vi "总磷总氮通讯.vi"() -> ()   [LabVIEW 2016, in "斯坦道总氮.lvlib"]
uses:
  <vilib>/Plasmionique/MB Master/MB_Master_Serial/MB_Master_Serial.lvclass
  C:/Program Files (x86)/National Instruments/LabVIEW 2016/vi.lib/Plasmionique/MB Master/MB_Master/MB_Master.lvclass
  <vilib>/Plasmionique/MB Master/MB_Master_TCP/MB_Master_TCP.lvclass
  <vilib>/Utility/config.llb/Write Key (Boolean).vi
  <vilib>/Utility/config.llb/Write Key (String).vi
  <vilib>/Plasmionique/MB Master/MB_Master/MB_Master.lvclass
  <vilib>/Utility/config.llb/NI_LVConfig.lvlib
  <vilib>/Plasmionique/MB Master/MB Master.lvlib
  <vilib>/ptbypt/NI_PtbyPt.lvlib
panel:
  out "启用":bool=TRUE
  out "氨氮状态告警区":u16[](array[numeric])
  out "氨氮测量数据区":u16[](array[numeric])
  out "COD测量数据区":u16[](array[numeric])
  out "COD状态告警区":u16[](array[numeric])
  out "总氮测量数据区":u16[](array[numeric])
  out "总氮状态告警区":u16[](array[numeric])
  out "总磷状态告警区":u16[](array[numeric])
  out "总磷测量数据区":u16[](array[numeric])
  out "状态告警区":T1 {"告警代码" items=["无告警", "缺试剂告警", "缺水样告警", "缺蒸馏水告警", "缺标液告警", "仪表漏液告警", "标定异常告警", "超量程告警", "加热异常", "低试剂预警", "超上限告警", "超下限告警", "仪表内部其他异常", "滴定异常告警", "电极异常告警", "量程切换告警", "参数设置告警", "PH电极电位异常", "电导率电极异常", "浊度光度异常", "溶解氧电极异常", "溶解氧光强异常", "温度异常告警", "PH异常告警", "溶解氧异常告警", "电导率异常告警", "浊度异常告警", "叶绿素异常告警", "藻密度异常告警", "蓝绿藻异常告警", "ORP异常告警", "氨氮异常告警", "清洁刷异常告警", "SD卡异常告警", "蓝牙异常告警", "Wifi异常告警", "流程异常告警"]; "故障代码" items=["无故障", "电机故障", "温度故障", "通讯故障", "滴定故障"]}
  out "测量数据区":T2 {"单位" items=["ug/L", "mg/L", "ppm", "mg/m3", "cm", "ppb", "ug/m3", "%", "nmol/mol", "umol/mol", "MPN/L", "MPN/100ml", "ng/m3", "NTU", "无量纲", "ms/cm", "us/cm", "℃", "mV", "万个/L"]}
  out "status":bool
  out "关键参数区":T3
  in  "读关键参数区":bool
  in  "读状态告警区":bool
  in  "读测量数据区":bool
  in  "站号":u16(ring) items=["总磷"=1, "氨氮"=3]
  in  "停止":bool
  in  "启动":bool
  in  "控制命令":u16(ring) items=["启动测量"=1, "标样核查"=2, "零点核查"=3, "跨度核查"=4, "空白测试"=5, "平行样测试"=6, "加标回收"=7, "空白校准"=8, "标样校准"=9, "初始化（清洗）"=10, "停止测试"=11, "仪器重启"=12, "校时"=13, "模式设置"=14, "测量间隔设置"=15]
  in  "控制命令参数":u16[](array[numeric]) format="%04xH"
  in  "VISA Resource":refnum<visa-resource-name>
  in  "启用模块":bool
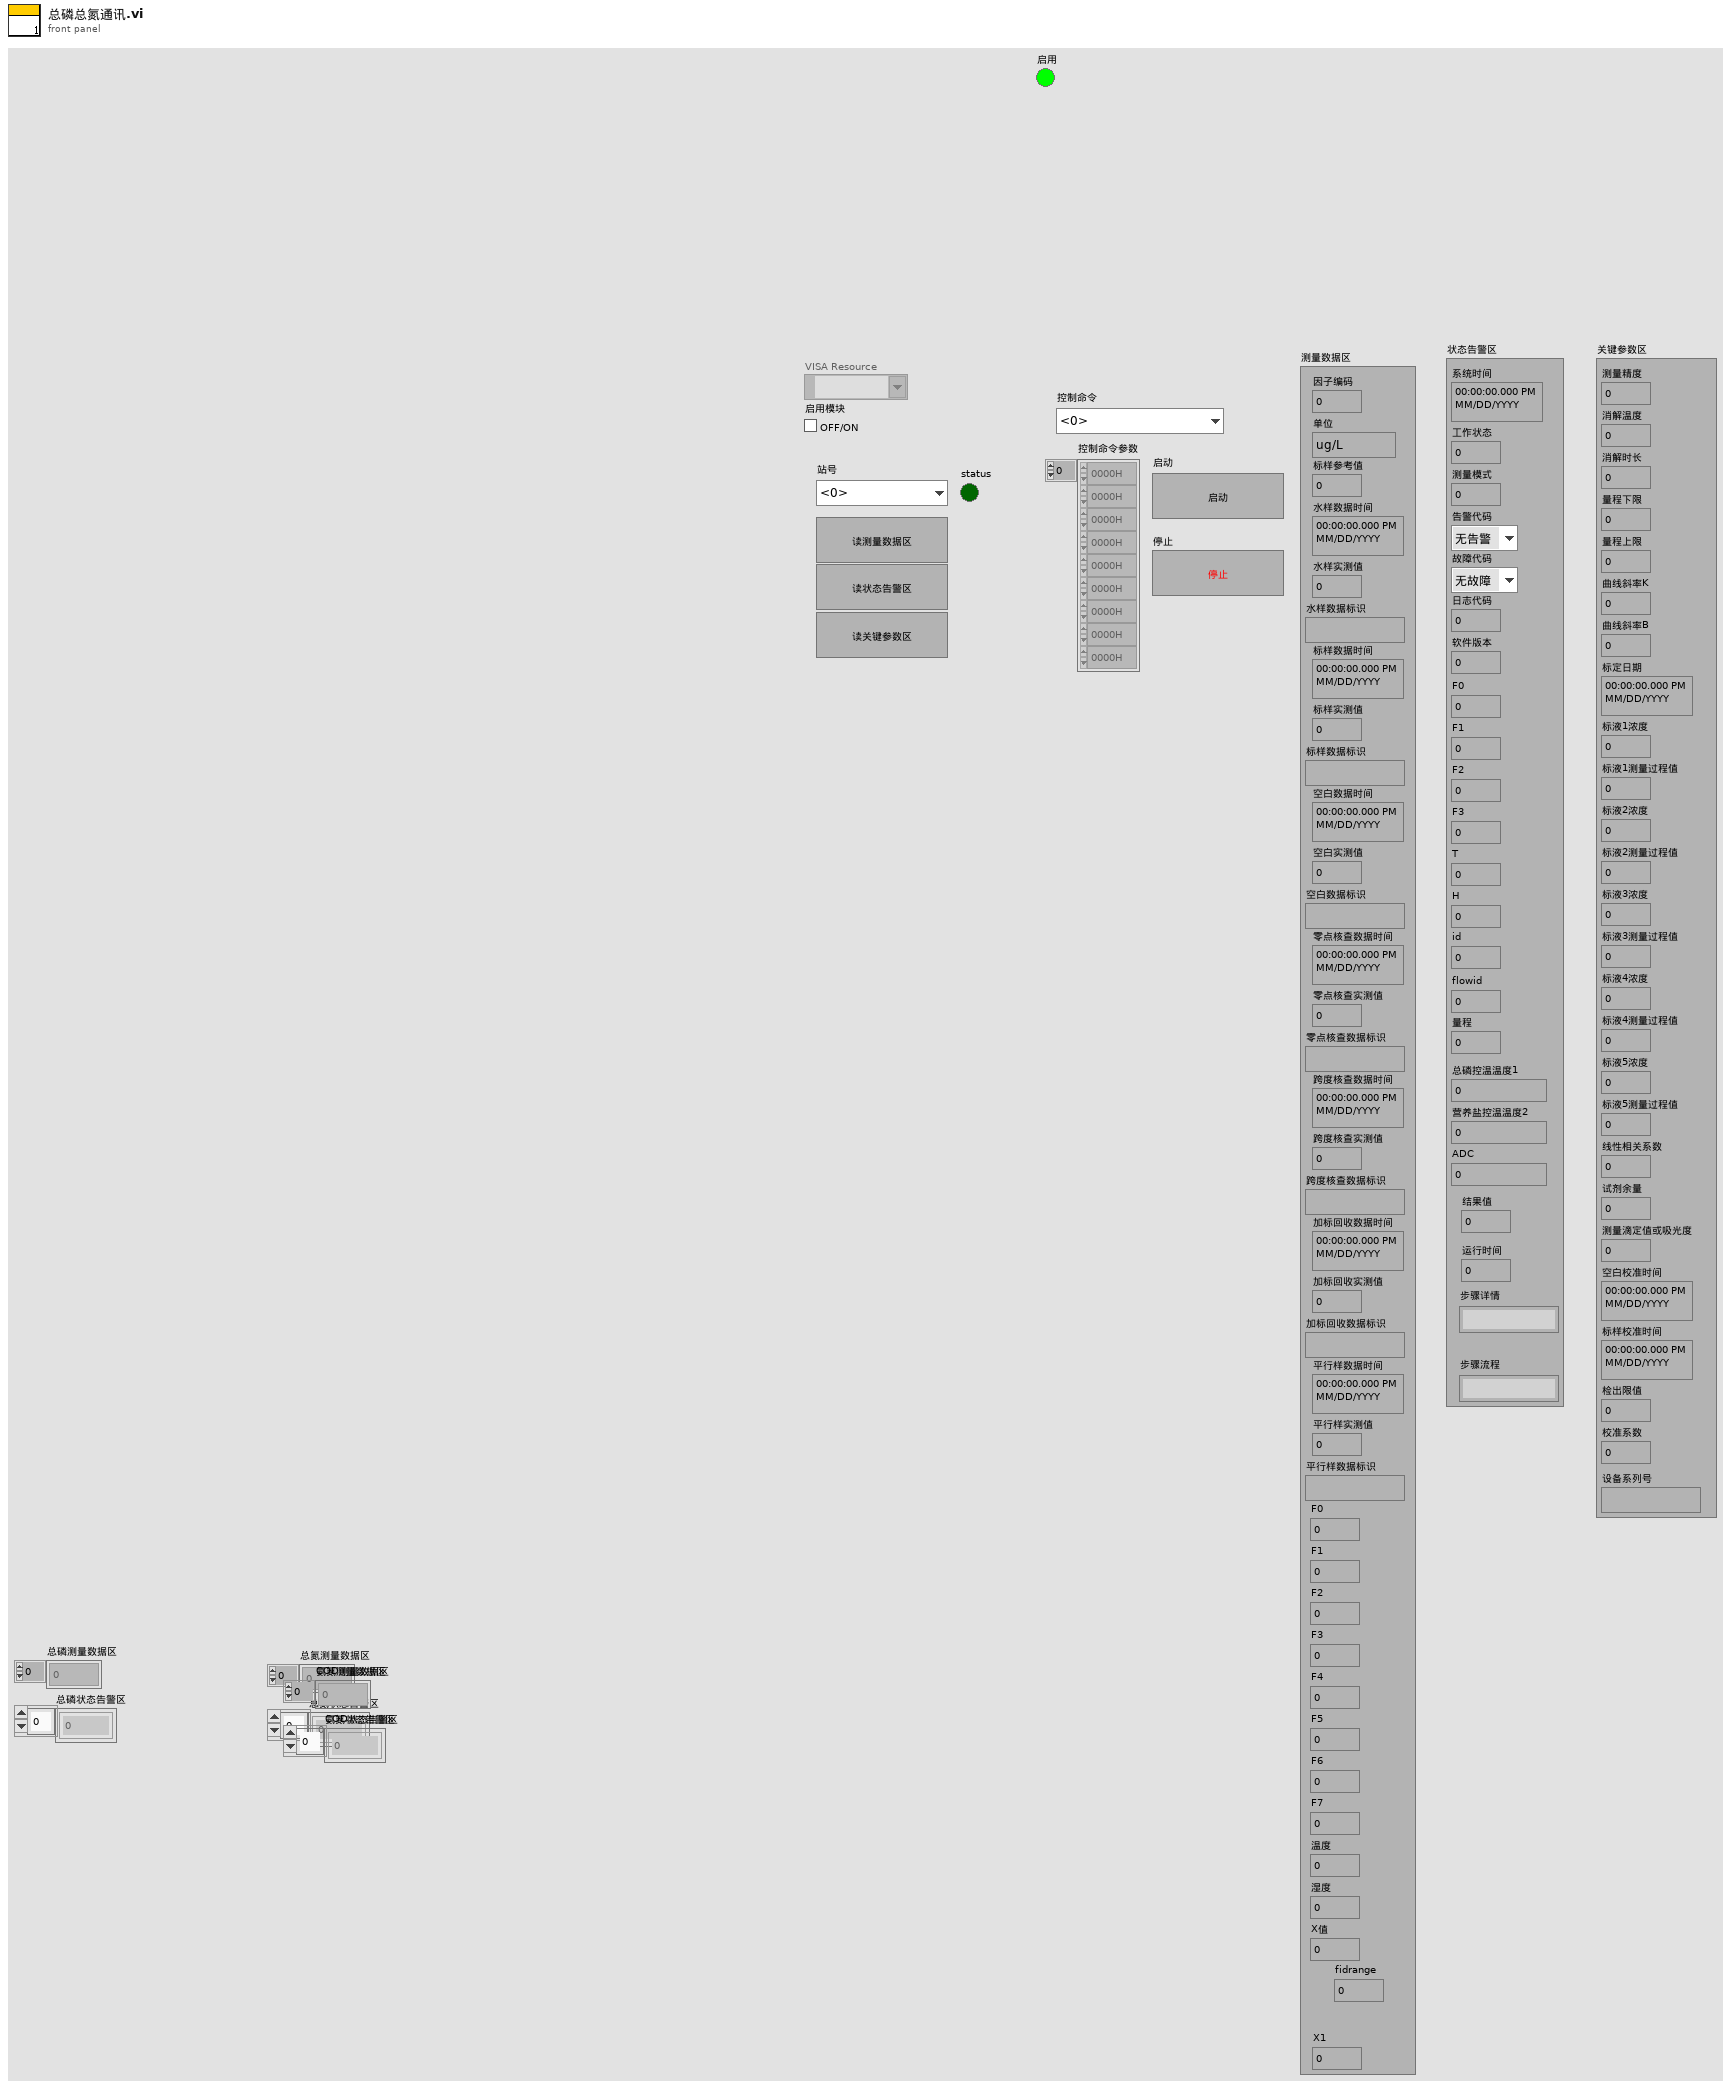
[diagram p1: front panel]
types:
  T1 = cluster{"系统时间":timestamp, "工作状态":u16, "测量模式":u16, "告警代码":u16, "故障代码":u16, "日志代码":u16, "软件版本":u16, "F0":sgl, "F1":sgl, "F2":sgl, "F3":sgl, "T":sgl, "H":sgl, "id":u16, "flowid":u16, "量程":u16, "总磷控温温度1":sgl, "营养盐控温温度2":sgl, "ADC":sgl, "结果值":sgl, "运行时间":u16, "步骤详情":string, "步骤流程":string}
  T2 = cluster{"因子编码":u32, "单位":u16, "标样参考值":sgl, "水样数据时间":timestamp, "水样实测值":sgl, "水样数据标识":string, "标样数据时间":timestamp, "标样实测值":sgl, "标样数据标识":string, "空白数据时间":timestamp, "空白实测值":sgl, "空白数据标识":string, "零点核查数据时间":timestamp, "零点核查实测值":sgl, "零点核查数据标识":string, "跨度核查数据时间":timestamp, "跨度核查实测值":sgl, "跨度核查数据标识":string, "加标回收数据时间":timestamp, "加标回收实测值":sgl, "加标回收数据标识":string, "平行样数据时间":timestamp, "平行样实测值":sgl, "平行样数据标识":string, "F0":sgl, "F1":sgl, "F2":sgl, "F3":sgl, "F4":sgl, "F5":sgl, "F6":sgl, "F7":sgl, "温度":sgl, "湿度":sgl, "X值":sgl, "fidrange":u16, "X1":sgl}
  T3 = cluster{"测量精度":u16, "消解温度":u16, "消解时长":u16, "量程下限":sgl, "量程上限":sgl, "曲线斜率K":sgl, "曲线斜率B":sgl, "标定日期":timestamp, "标液1浓度":sgl, "标液1测量过程值":sgl, "标液2浓度":sgl, "标液2测量过程值":sgl, "标液3浓度":sgl, "标液3测量过程值":sgl, "标液4浓度":sgl, "标液4测量过程值":sgl, "标液5浓度":sgl, "标液5测量过程值":sgl, "线性相关系数":sgl, "试剂余量":u32, "测量滴定值或吸光度":sgl, "空白校准时间":timestamp, "标样校准时间":timestamp, "检出限值":sgl, "校准系数":sgl, "设备系列号":string}
  T4 = cluster{"系统时间":timestamp, "工作状态":u16, "测量模式":enum16{"待机", "连续模式", "周期模式", "定点模式", "受控模式", "手动模式"}, "告警代码":u16, "故障代码":u16, "日志代码":u16, "软件版本":u16, "F0":sgl, "F1":sgl, "F2":sgl, "F3":sgl, "T":sgl, "H":sgl, "id":u16, "flowid":u16, "量程":u16, "总磷控温温度1":sgl, "营养盐控温温度2":sgl, "ADC":sgl}
  T5 = cluster{"因子编码":u32, "单位":u16, "标样参考值":sgl, "水样数据时间":timestamp, "水样实测值":sgl, "水样数据标识":string, "标样数据时间":timestamp, "标样实测值":sgl, "标样数据标识":string, "空白数据时间":timestamp, "空白实测值":sgl, "空白数据标识":string, "零点核查数据时间":timestamp, "零点核查实测值":sgl, "零点核查数据标识":string, "跨度核查数据时间":timestamp, "跨度核查实测值":sgl, "跨度核查数据标识":string, "加标回收数据时间":timestamp, "加标回收实测值":sgl, "加标回收数据标识":string, "平行样数据时间":timestamp, "平行样实测值":sgl, "平行样数据标识":string, "F0":sgl, "F1":sgl, "F2":sgl, "F3":sgl, "F4":sgl, "F5":sgl, "F6":sgl, "F7":sgl, "温度":sgl, "湿度":sgl, "X值":sgl, "fidrange":u16, "X1值":sgl}
  T6 = cluster{"测量精度":u16, "消解温度":u16, "消解时长":u16, "量程下限":sgl, "量程上限":sgl, "曲线斜率K":sgl, "曲线斜率B":sgl, "标定日期":timestamp, "标液1浓度":sgl, "标液1测量过程值":sgl, "标液2浓度":sgl, "标液2测量过程值":sgl, "标液3浓度":sgl, "标液3测量过程值":sgl, "标液4浓度":sgl, "标液4测量过程值":sgl, "标液5浓度":sgl, "标液5测量过程值":sgl, "线性相关系数":sgl, "试剂余量":u32, "测量滴定值或吸光度":sgl, "空白校准时间":timestamp, "标样校准时间":timestamp, "检出限值":sgl, "校准系数":sgl, "设备系列号":string}[]
  T7 = cluster{"系统时间":timestamp, "工作状态":u16, "测量模式":enum16{"待机", "连续模式", "周期模式", "定点模式", "受控模式", "手动模式"}, "告警代码":u16, "故障代码":u16, "日志代码":u16, "软件版本":u16, "F0":sgl, "F1":sgl, "F2":sgl, "F3":sgl, "T":sgl, "H":sgl, "id":u16, "flowid":u16, "量程":u16, "总磷控温温度1":sgl, "营养盐控温温度2":sgl, "ADC":sgl}[]
  T8 = cluster{"因子编码":u32, "单位":u16, "标样参考值":sgl, "水样数据时间":timestamp, "水样实测值":sgl, "水样数据标识":string, "标样数据时间":timestamp, "标样实测值":sgl, "标样数据标识":string, "空白数据时间":timestamp, "空白实测值":sgl, "空白数据标识":string, "零点核查数据时间":timestamp, "零点核查实测值":sgl, "零点核查数据标识":string, "跨度核查数据时间":timestamp, "跨度核查实测值":sgl, "跨度核查数据标识":string, "加标回收数据时间":timestamp, "加标回收实测值":sgl, "加标回收数据标识":string, "平行样数据时间":timestamp, "平行样实测值":sgl, "平行样数据标识":string, "F0":sgl, "F1":sgl, "F2":sgl, "F3":sgl, "F4":sgl, "F5":sgl, "F6":sgl, "F7":sgl, "温度":sgl, "湿度":sgl, "X值":sgl, "fidrange":u16, "X1值":sgl}[]
  T9 = enum16{"", "CODMn", "PH", "氨氮", "总氮", "总磷", "CODCr", "电导率", "水温", "溶解氧", "浊度", "叶绿素", "藻密度", "ORP"}
  T10 = typedef "CODCr交互.ctl" = cluster{"状态告警区":cluster{"系统时间":timestamp, "工作状态":u16, "测量模式":enum16{"待机", "连续模式", "周期模式", "定点模式", "受控模式", "手动模式"}, "告警代码":u16, "故障代码":u16, "日志代码":u16, "软件版本":u16, "F0":sgl, "F1":sgl, "F2":sgl, "F3":sgl, "T":sgl, "H":sgl, "id":u16, "flowid":u16, "量程":u16, "总磷控温温度1":sgl, "营养盐控温温度2":sgl, "ADC":sgl}, "平台试剂余量百分比":sgl, "关键参数":cluster{"测量量程":dbl, "测量精度":dbl, "测量间隔":dbl, "消解温度":dbl, "消解时长":dbl, "空白校准时间":timestamp, "曲线截距":dbl, "曲线斜率":dbl, "测量检出限":dbl, "测量信号值":dbl, "线性相关系数":dbl, "二次多项式系数":dbl, "标样校准时间":timestamp, "稀释倍数":dbl, "三项式系数":dbl, "空白标定系数":dbl, "量程系数":dbl, "F0/ORPA":dbl, "F1/ORPB":dbl, "F2/ORPK":dbl, "F3":dbl, "F4":dbl, "F5":dbl, "F6":dbl, "F7":dbl, "X0/滴定数":dbl, "量程":dbl}, "关键参数改变":bool, "校准信息":cluster{"低标液1浓度":dbl, "低标液1信号值":dbl, "低标液1启用":u16, "低标液2浓度":dbl, "低标液2信号值":dbl, "低标液2启用":u16, "低标液3浓度":dbl, "低标液3信号值":dbl, "低标液3启用":u16, "低标液4浓度":dbl, "低标液4信号值":dbl, "低标液4启用":u16, "低标液5浓度":dbl, "低标液5信号值":dbl, "低标液5启用":u16, "高标液1浓度":dbl, "高标液1信号值":dbl, "高标液1启用":u16, "高标液2浓度":dbl, "高标液2信号值":dbl, "高标液2启用":u16, "高标液3浓度":dbl, "高标液3信号值":dbl, "高标液3启用":u16, "高标液4浓度":dbl, "高标液4信号值":dbl, "高标液4启用":u16, "高标液5浓度":dbl, "高标液5信号值":dbl, "高标液5启用":u16, "低斜率":dbl, "低截距":dbl, "低二次多项式系数":dbl, "低线性相关系数":dbl, "高斜率":dbl, "高截距":dbl, "高二次多项式系数":dbl, "高线性相关系数":dbl}, "校准信息改变":bool, "固件版本号":string}
  T11 = typedef "氨氮交互.ctl" = cluster{"状态告警区":cluster{"系统时间":timestamp, "工作状态":u16, "测量模式":enum16{"待机", "连续模式", "周期模式", "定点模式", "受控模式", "手动模式"}, "告警代码":u16, "故障代码":u16, "日志代码":u16, "软件版本":u16, "F0":sgl, "F1":sgl, "F2":sgl, "F3":sgl, "T":sgl, "H":sgl, "id":u16, "flowid":u16, "量程":u16, "总磷控温温度1":sgl, "营养盐控温温度2":sgl, "ADC":sgl}, "平台试剂余量百分比":sgl, "关键参数":cluster{"测量量程":dbl, "测量精度":dbl, "测量间隔":dbl, "消解温度":dbl, "消解时长":dbl, "空白校准时间":timestamp, "曲线截距":dbl, "曲线斜率":dbl, "测量检出限":dbl, "测量信号值":dbl, "线性相关系数":dbl, "二次多项式系数":dbl, "标样校准时间":timestamp, "稀释倍数":dbl, "三项式系数":dbl, "空白标定系数":dbl, "量程系数":dbl, "F0/ORPA":dbl, "F1/ORPB":dbl, "F2/ORPK":dbl, "F3":dbl, "F4":dbl, "F5":dbl, "F6":dbl, "F7":dbl, "X0/滴定数":dbl, "量程":dbl}, "关键参数改变":bool, "校准信息":cluster{"低标液1浓度":dbl, "低标液1信号值":dbl, "低标液1启用":u16, "低标液2浓度":dbl, "低标液2信号值":dbl, "低标液2启用":u16, "低标液3浓度":dbl, "低标液3信号值":dbl, "低标液3启用":u16, "低标液4浓度":dbl, "低标液4信号值":dbl, "低标液4启用":u16, "低标液5浓度":dbl, "低标液5信号值":dbl, "低标液5启用":u16, "高标液1浓度":dbl, "高标液1信号值":dbl, "高标液1启用":u16, "高标液2浓度":dbl, "高标液2信号值":dbl, "高标液2启用":u16, "高标液3浓度":dbl, "高标液3信号值":dbl, "高标液3启用":u16, "高标液4浓度":dbl, "高标液4信号值":dbl, "高标液4启用":u16, "高标液5浓度":dbl, "高标液5信号值":dbl, "高标液5启用":u16, "低斜率":dbl, "低截距":dbl, "低二次多项式系数":dbl, "低线性相关系数":dbl, "高斜率":dbl, "高截距":dbl, "高二次多项式系数":dbl, "高线性相关系数":dbl}, "校准信息改变":bool, "固件版本号":string}
  T12 = typedef "总氮交互.ctl" = cluster{"状态告警区":cluster{"系统时间":timestamp, "工作状态":u16, "测量模式":enum16{"待机", "连续模式", "周期模式", "定点模式", "受控模式", "手动模式"}, "告警代码":u16, "故障代码":u16, "日志代码":u16, "软件版本":u16, "F0":sgl, "F1":sgl, "F2":sgl, "F3":sgl, "T":sgl, "H":sgl, "id":u16, "flowid":u16, "量程":u16, "总磷控温温度1":sgl, "营养盐控温温度2":sgl, "ADC":sgl}, "平台试剂余量百分比":sgl, "关键参数":cluster{"测量量程":dbl, "测量精度":dbl, "测量间隔":dbl, "消解温度":dbl, "消解时长":dbl, "空白校准时间":timestamp, "曲线截距":dbl, "曲线斜率":dbl, "测量检出限":dbl, "测量信号值":dbl, "线性相关系数":dbl, "二次多项式系数":dbl, "标样校准时间":timestamp, "稀释倍数":dbl, "三项式系数":dbl, "空白标定系数":dbl, "量程系数":dbl, "F0/ORPA":dbl, "F1/ORPB":dbl, "F2/ORPK":dbl, "F3":dbl, "F4":dbl, "F5":dbl, "F6":dbl, "F7":dbl, "X0/滴定数":dbl, "量程":dbl}, "关键参数改变":bool, "校准信息":cluster{"低标液1浓度":dbl, "低标液1信号值":dbl, "低标液1启用":u16, "低标液2浓度":dbl, "低标液2信号值":dbl, "低标液2启用":u16, "低标液3浓度":dbl, "低标液3信号值":dbl, "低标液3启用":u16, "低标液4浓度":dbl, "低标液4信号值":dbl, "低标液4启用":u16, "低标液5浓度":dbl, "低标液5信号值":dbl, "低标液5启用":u16, "高标液1浓度":dbl, "高标液1信号值":dbl, "高标液1启用":u16, "高标液2浓度":dbl, "高标液2信号值":dbl, "高标液2启用":u16, "高标液3浓度":dbl, "高标液3信号值":dbl, "高标液3启用":u16, "高标液4浓度":dbl, "高标液4信号值":dbl, "高标液4启用":u16, "高标液5浓度":dbl, "高标液5信号值":dbl, "高标液5启用":u16, "低斜率":dbl, "低截距":dbl, "低二次多项式系数":dbl, "低线性相关系数":dbl, "高斜率":dbl, "高截距":dbl, "高二次多项式系数":dbl, "高线性相关系数":dbl}, "校准信息改变":bool, "固件版本号":string}
  T13 = typedef "总磷交互.ctl" = cluster{"状态告警区":cluster{"系统时间":timestamp, "工作状态":u16, "测量模式":enum16{"待机", "连续模式", "周期模式", "定点模式", "受控模式", "手动模式"}, "告警代码":u16, "故障代码":u16, "日志代码":u16, "软件版本":u16, "F0":sgl, "F1":sgl, "F2":sgl, "F3":sgl, "T":sgl, "H":sgl, "id":u16, "flowid":u16, "量程":u16, "总磷控温温度1":sgl, "营养盐控温温度2":sgl, "ADC":sgl}, "平台试剂余量百分比":sgl, "关键参数":cluster{"测量量程":dbl, "测量精度":dbl, "测量间隔":dbl, "消解温度":dbl, "消解时长":dbl, "空白校准时间":timestamp, "曲线截距":dbl, "曲线斜率":dbl, "测量检出限":dbl, "测量信号值":dbl, "线性相关系数":dbl, "二次多项式系数":dbl, "标样校准时间":timestamp, "稀释倍数":dbl, "三项式系数":dbl, "空白标定系数":dbl, "量程系数":dbl, "F0/ORPA":dbl, "F1/ORPB":dbl, "F2/ORPK":dbl, "F3":dbl, "F4":dbl, "F5":dbl, "F6":dbl, "F7":dbl, "X0/滴定数":dbl, "量程":dbl}, "关键参数改变":bool, "校准信息":cluster{"低标液1浓度":dbl, "低标液1信号值":dbl, "低标液1启用":u16, "低标液2浓度":dbl, "低标液2信号值":dbl, "低标液2启用":u16, "低标液3浓度":dbl, "低标液3信号值":dbl, "低标液3启用":u16, "低标液4浓度":dbl, "低标液4信号值":dbl, "低标液4启用":u16, "低标液5浓度":dbl, "低标液5信号值":dbl, "低标液5启用":u16, "高标液1浓度":dbl, "高标液1信号值":dbl, "高标液1启用":u16, "高标液2浓度":dbl, "高标液2信号值":dbl, "高标液2启用":u16, "高标液3浓度":dbl, "高标液3信号值":dbl, "高标液3启用":u16, "高标液4浓度":dbl, "高标液4信号值":dbl, "高标液4启用":u16, "高标液5浓度":dbl, "高标液5信号值":dbl, "高标液5启用":u16, "低斜率":dbl, "低截距":dbl, "低二次多项式系数":dbl, "低线性相关系数":dbl, "高斜率":dbl, "高截距":dbl, "高二次多项式系数":dbl, "高线性相关系数":dbl}, "校准信息改变":bool, "固件版本号":string}
  T14 = typedef "操作日志字段定义.ctl" = cluster{"时间":timestamp, "参数":string, "日志信息":string, "流程参数":string}
  T15 = typedef "NI_LVConfig.lvlib/Config Data RefNum.ctl" = refnum<k1>
  T16 = enum8{"Enabled", "Disabled", "Disabled and Grayed Out"}
  T17 = cluster{"baud rate (bps)":u32, "stop bits":u16, "parity":u16, "flow control":u16, "timeout":u32, "retries":i32}
  T18 = typedef "工况数据.ctl" = cluster{"time":string, "data":cluster{"ups":cluster{"ups":cluster{"input_voltage":ext, "input_frequency":ext, "output_voltage":ext, "output_current":ext, "output_frequency":ext, "output_active_power":ext, "output_apparent_power":ext, "load_rate":ext, "cabinet_temperature":ext, "battery_voltage":ext, "remaining_battery_capacity":ext, "power_on_status":string, "power_supply_mode":string, "fault":bool, "battery_low_voltage":bool, "mains_supply_abnormality":bool}, "启用":bool}, "air_conditioner":cluster{"air_conditioner":cluster{"cabinet_temperature":ext, "air_supply_temperature":ext, "voltage":ext, "current":ext, "compressor_status":string, "Internal_fan_status":string, "external_fan_status":string, "heating_state":string, "refrigeration_state":bool, "high_temperature_alarm":bool, "low_temperature_alarm":bool, "heater_fault":bool, "temperature_sensor_fault":bool, "high_voltage_alarm":bool, "low_voltage_alarm":bool, "refrigeration_start_point":ext, "refrigeration_sensitive_point":ext, "heating_start_point":ext, "heating_sensitive_point":ext, "high_temperature_alarm_point":ext, "low_temperature_alarm_point":ext}, "启用":bool}, "smoke_sensor":cluster{"smoke_sensor":cluster{"trigger_alarm":bool}, "启用":bool}, "water_immersion_sensor":cluster{"water_immersion_sensor":cluster{"trigger_alarm":bool}, "启用":bool}, "temperature_and_humidity_sensor":cluster{"temperature_and_humidity_sensor":cluster{"current_temperature":ext, "current_humidity":ext, "room_temperature_alarm":bool, "humidity_alarm":bool}, "启用":bool}, "gps":cluster{"gps":cluster{"current_longitude":ext, "current_latitude":ext, "launch_longitude":ext, "launch_latitude":ext, "shift_alarm":bool}, "启用":bool}, "solar_controller":cluster{"solar_controller":cluster{"array_voltage":ext, "array_current":ext, "generating_power":ext, "battery_voltage":dbl, "battery_current":ext, "ceiling_voltage":ext, "minimum_voltage":ext, "battery_temperature":ext, "remaining_battery_capacity":ext, "load_voltage":ext, "load_current":ext, "load_power":ext, "equipment_temperature":ext, "accumulated_electricity_consumption_of_the_day":ext, "accumulated_electricity_consumption_of_the_current_month":ext, "accumulated_electricity_consumption_in_the_current_year":ext, "total_accumulated_power_consumption":ext, "accumulated_charging_capacity_of_the_day":ext, "accumulated_charging_amount_of_the_current_month":ext, "accumulated_charging_capacity_of_the_current_year":ext, "total_cumulative_charge":ext}, "启用":bool}, "solar_controller_2":cluster{"solar_controller_2":cluster{"array_voltage":ext, "array_current":ext, "generating_power":ext, "battery_voltage":dbl, "battery_current":ext, "ceiling_voltage":ext, "minimum_voltage":ext, "battery_temperature":ext, "remaining_battery_capacity":ext, "load_voltage":ext, "load_current":ext, "load_power":ext, "equipment_temperature":ext, "accumulated_electricity_consumption_of_the_day":ext, "accumulated_electricity_consumption_of_the_current_month":ext, "accumulated_electricity_consumption_in_the_current_year":ext, "total_accumulated_power_consumption":ext, "accumulated_charging_capacity_of_the_day":ext, "accumulated_charging_amount_of_the_current_month":ext, "accumulated_charging_capacity_of_the_current_year":ext, "total_cumulative_charge":ext}, "启用":bool}, "NH3":cluster{"NH3":cluster{"F0":ext, "F1":ext, "syringe_temperature":ext, "alarm_step":dbl, "X0":ext}, "启用":bool}, "TP":cluster{"TP":cluster{"F0":ext, "F1":ext, "F2":ext, "F3":ext, "digestion_temperature":ext, "constant_temperature":ext, "syringe_temperature":ext, "alarm_step":dbl, "X0":ext}, "启用":bool}, "TN":cluster{"TN":cluster{"F0":ext, "F1":ext, "F2":ext, "F3":ext, "F4":ext, "F5":ext, "F6":ext, "F7":ext, "digestion_temperature":ext, "constant_temperature":ext, "syringe_temperature":ext, "alarm_step":dbl, "X0":ext}, "启用":bool}, "CODMn":cluster{"CODMn":cluster{"temperature_curve":ext[], "titration_curve":ext[], "F0":ext, "F1":ext, "F2":ext, "F3":ext, "F4":ext, "F5":ext, "A":ext, "B":ext, "K":ext}, "启用":bool}, "CODCr":cluster{"CODCr":cluster{"temperature_curve":ext[], "F0":ext, "F1":ext, "reagent_sensor":ext}, "启用":bool}}}
  T19 = cluster{"系统时间":timestamp, "工作状态":u16, "测量模式":enum16{"待机", "连续模式", "周期模式", "定点模式", "受控模式", "手动模式"}, "告警代码":u16, "故障代码":u16, "日志代码":u16, "软件版本":u16, "F0":sgl, "F1":sgl, "F2":sgl, "F3":sgl, "T":sgl, "H":sgl, "id":u16, "flowid":u16, "量程":u16, "总磷控温温度1":sgl, "营养盐控温温度2":sgl, "ADC":sgl, "结果值":sgl, "运行时间":u16, "步骤详情":string, "步骤流程":string}
  T20 = typedef "斯坦道总氮.lvlib/关键参数.ctl" = cluster{"测量量程":sgl, "测量检出限":sgl, "测量精度":sgl, "测量间隔":sgl, "消解温度":sgl, "消解时长":sgl, "三项式系数":sgl, "二次多项式系数":sgl, "曲线斜率":sgl, "曲线截距":sgl, "线性相关系数":sgl, "空白校准时间":timestamp, "标样校准时间":timestamp, "测量信号值":sgl, "稀释倍数":sgl, "空白标定系数":sgl, "量程系数":sgl}
  T21 = cluster{"测量量程":dbl, "测量精度":dbl, "测量间隔":dbl, "消解温度":dbl, "消解时长":dbl, "空白校准时间":timestamp, "曲线截距":dbl, "曲线斜率":dbl, "测量检出限":dbl, "测量信号值":dbl, "线性相关系数":dbl, "二次多项式系数":dbl, "标样校准时间":timestamp, "稀释倍数":dbl, "三项式系数":dbl, "空白标定系数":dbl, "量程系数":dbl, "F0/ORPA":dbl, "F1/ORPB":dbl, "F2/ORPK":dbl, "F3":dbl, "F4":dbl, "F5":dbl, "F6":dbl, "F7":dbl, "X0/滴定数":dbl, "量程":dbl}
  T22 = cluster{"低标液1浓度":dbl, "低标液1信号值":dbl, "低标液1启用":u16, "低标液2浓度":dbl, "低标液2信号值":dbl, "低标液2启用":u16, "低标液3浓度":dbl, "低标液3信号值":dbl, "低标液3启用":u16, "低标液4浓度":dbl, "低标液4信号值":dbl, "低标液4启用":u16, "低标液5浓度":dbl, "低标液5信号值":dbl, "低标液5启用":u16, "高标液1浓度":dbl, "高标液1信号值":dbl, "高标液1启用":u16, "高标液2浓度":dbl, "高标液2信号值":dbl, "高标液2启用":u16, "高标液3浓度":dbl, "高标液3信号值":dbl, "高标液3启用":u16, "高标液4浓度":dbl, "高标液4信号值":dbl, "高标液4启用":u16, "高标液5浓度":dbl, "高标液5信号值":dbl, "高标液5启用":u16, "低斜率":dbl, "低截距":dbl, "低二次多项式系数":dbl, "低线性相关系数":dbl, "高斜率":dbl, "高截距":dbl, "高二次多项式系数":dbl, "高线性相关系数":dbl}
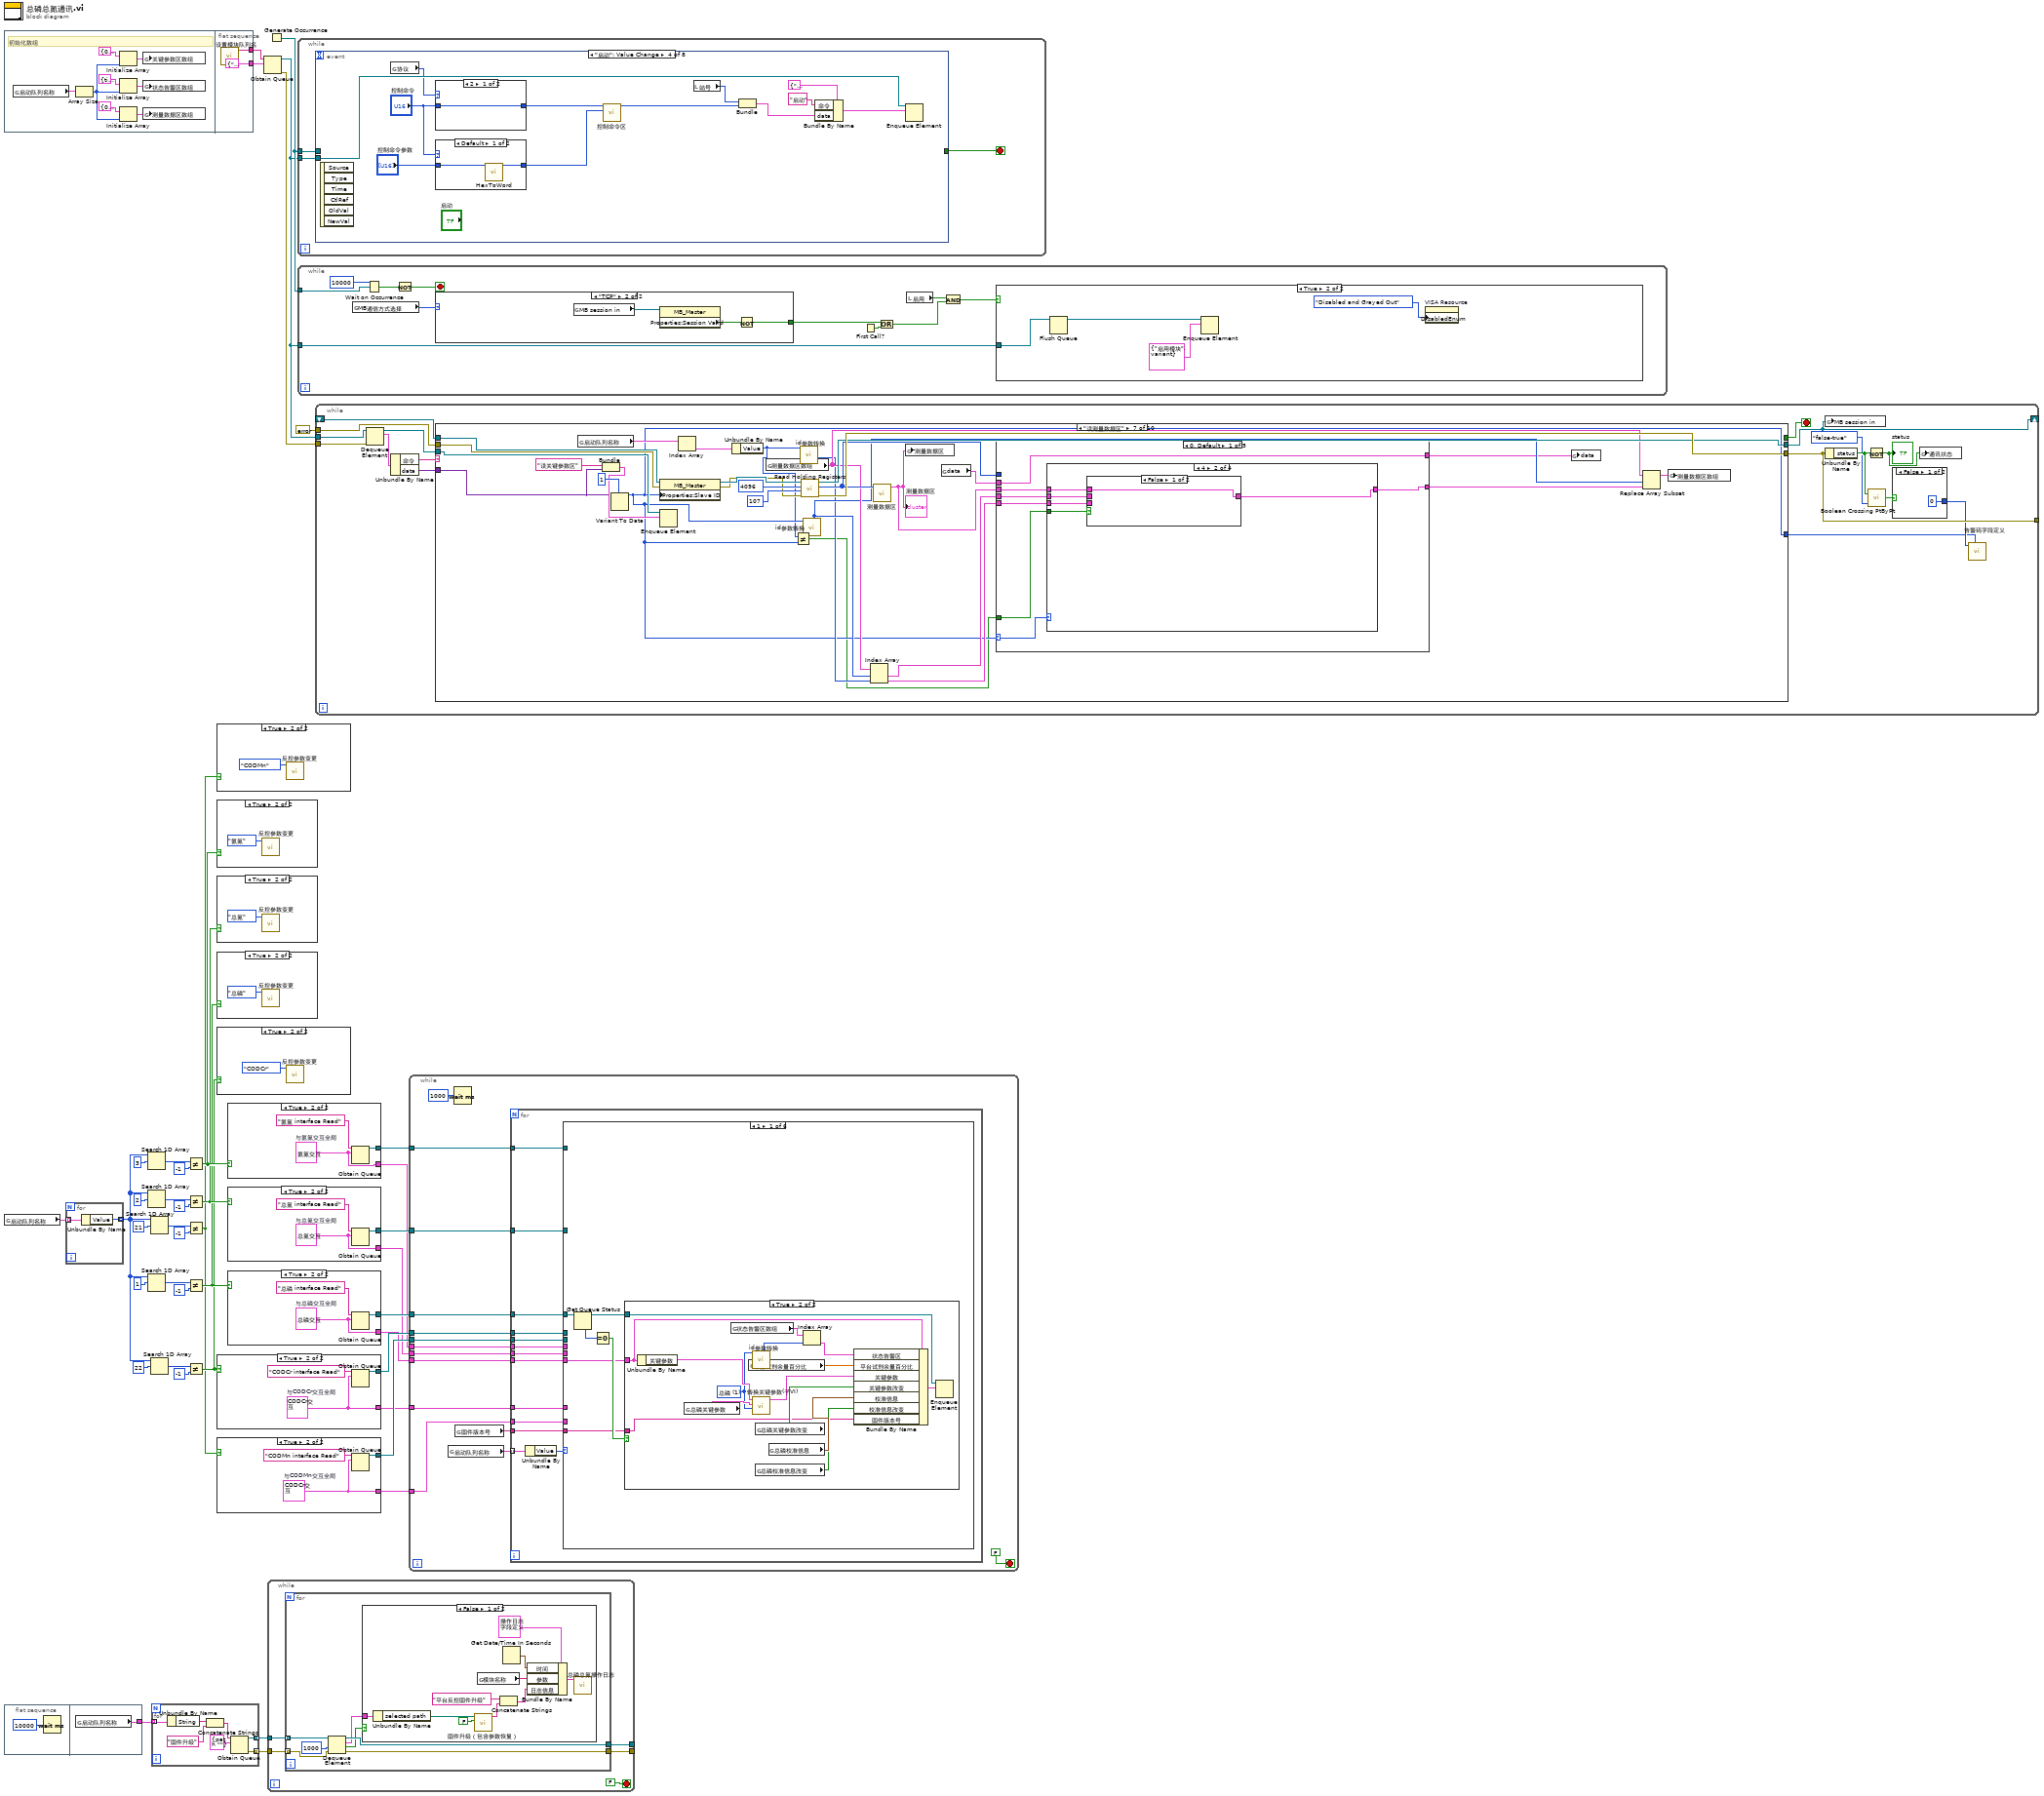
[diagram p0: block diagram]
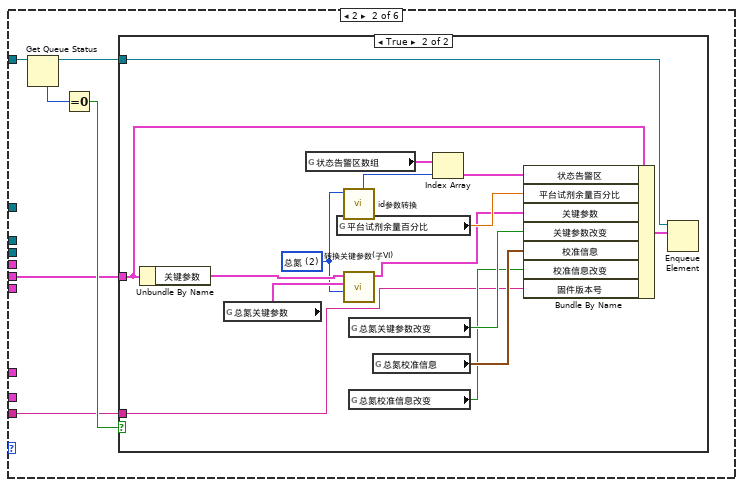
[diagram p14: hidden frame]
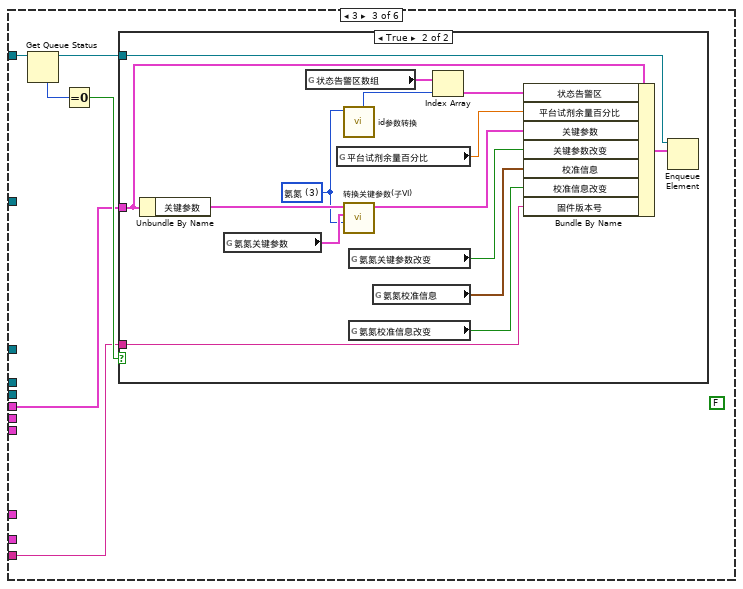
[diagram p16: hidden frame]
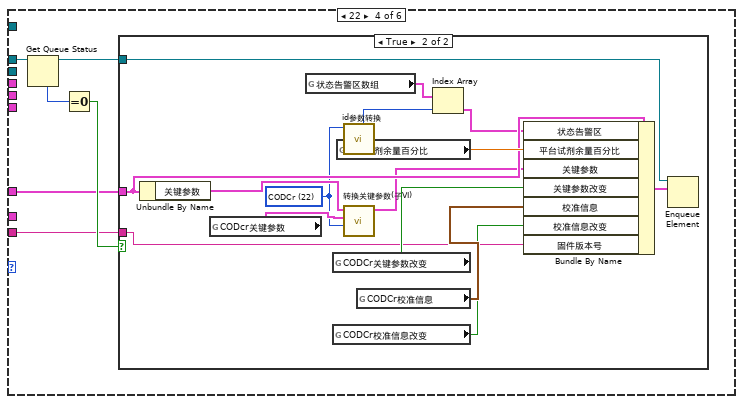
[diagram p18: hidden frame]
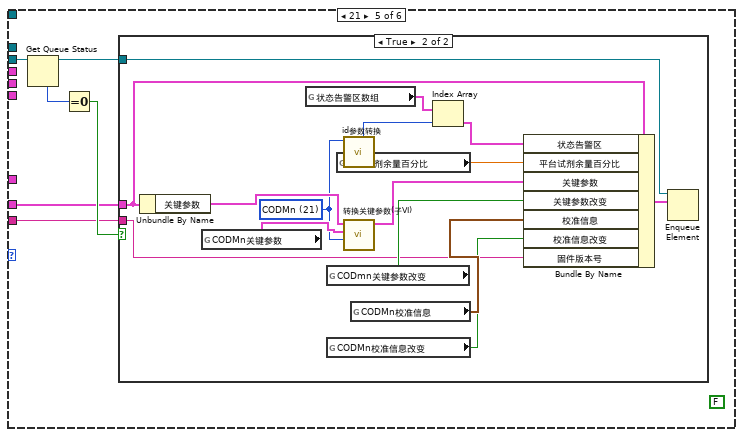
[diagram p20: hidden frame]
diagram:
  n1 = flat-sequence {
    tunnel: [cluster{"命令":string, "data":variant} {"命令"="", "data"=variant}] -> w41
    tunnel: [w50] -> w36
    frame #0 {
      # "初始化数组"
      n2 = global read "model config var.vi" "启动队列名称"() -> (w43:cluster{"String":string, "Value":u16}[])
      n3 = Array Size(array=w43) -> (size(s)=w42:i32)
      n4 = Initialize Array(T3 {"测量精度"=0, "消解温度"=0, "消解时长"=0, "量程下限"=0.0, "量程上限"=0.0, "曲线斜率K"=0.0, "曲线斜率B"=0.0, "标定日期"=timestamp(0 s since 1904-01-01), "标液1浓度"=0.0, "标液1测量过程值"=0.0, "标液2浓度"=0.0, "标液2测量过程值"=0.0, "标液3浓度"=0.0, "标液3测量过程值"=0.0, "标液4浓度"=0.0, "标液4测量过程值"=0.0, "标液5浓度"=0.0, "标液5测量过程值"=0.0, "线性相关系数"=0.0, "试剂余量"=0, "测量滴定值或吸光度"=0.0, "空白校准时间"=timestamp(0 s since 1904-01-01), "标样校准时间"=timestamp(0 s since 1904-01-01), "检出限值"=0.0, "校准系数"=0.0, "设备系列号"=""} ("关键参数区"), w42) -> (w47:T6)
      n5 = Initialize Array(T4 {"系统时间"=timestamp(0 s since 1904-01-01), "工作状态"=0, "测量模式"=enum."待机", "告警代码"=0, "故障代码"=0, "日志代码"=0, "软件版本"=0, "F0"=0.0, "F1"=0.0, "F2"=0.0, "F3"=0.0, "T"=0.0, "H"=0.0, "id"=0, "flowid"=0, "量程"=0, "总磷控温温度1"=0.0, "营养盐控温温度2"=0.0, "ADC"=0.0} ("状态告警区"), w42) -> (w46:T7)
      n6 = Initialize Array(T5 {"因子编码"=0, "单位"=0, "标样参考值"=0.0, "水样数据时间"=timestamp(0 s since 1904-01-01), "水样实测值"=0.0, "水样数据标识"="", "标样数据时间"=timestamp(0 s since 1904-01-01), "标样实测值"=0.0, "标样数据标识"="", "空白数据时间"=timestamp(0 s since 1904-01-01), "空白实测值"=0.0, "空白数据标识"="", "零点核查数据时间"=timestamp(0 s since 1904-01-01), "零点核查实测值"=0.0, "零点核查数据标识"="", "跨度核查数据时间"=timestamp(0 s since 1904-01-01), "跨度核查实测值"=0.0, "跨度核查数据标识"="", "加标回收数据时间"=timestamp(0 s since 1904-01-01), "加标回收实测值"=0.0, "加标回收数据标识"="", "平行样数据时间"=timestamp(0 s since 1904-01-01), "平行样实测值"=0.0, "平行样数据标识"="", "F0"=0.0, "F1"=0.0, "F2"=0.0, "F3"=0.0, "F4"=0.0, "F5"=0.0, "F6"=0.0, "F7"=0.0, "温度"=0.0, "湿度"=0.0, "X值"=0.0, "fidrange"=0, "X1值"=0.0} ("测量数据区"), w42) -> (w49:T8)
      n7 = global write "VAR总磷总氮全局变量.vi" "关键参数区数组"(w47) -> ()
      n8 = global write "VAR总磷总氮全局变量.vi" "状态告警区数组"(w46) -> ()
      n9 = global write "VAR总磷总氮全局变量.vi" "测量数据区数组"(w49) -> ()
    }
    frame #1 {
      n10 = call "设置模块队列名.vi"() -> ("Msg"=w50:string)  [unwired: 5 in]
    }
  }
  n11 = global read "model config var.vi" "启动队列名称"() -> (w25:cluster{"String":string, "Value":u16}[])
  n12 = flat-sequence {
    tunnel: [w53] -> w8
    frame #0 {
      n13 = Wait (ms)(milliseconds to wait=u32 10000 ("等待时间（毫秒）")) -> ()  [unwired: 1 out]
    }
    frame #1 {
      n14 = global read "model config var.vi" "启动队列名称"() -> (w53:cluster{"String":string, "Value":u16}[])
    }
  }
  n15 = for {
    tunnel: w25 -> [w55] mode=indexing
    tunnel: [w54] -> w9 mode=indexing
    n16 = Unbundle By Name(w55) -> ("Value"=w54:u16)
  }
  n17 = Search 1D Array(1D array=w9, element=u16 3 ("元素")) -> (index of element=w11:i32)  [unwired: 1 in]
  n18 = Search 1D Array(1D array=w9, element=u16 2 ("元素")) -> (index of element=w14:i32)  [unwired: 1 in]
  n19 = Search 1D Array(1D array=w9, element=u16 1 ("元素")) -> (index of element=w17:i32)  [unwired: 1 in]
  n20 = Search 1D Array(1D array=w9, element=u16 21 ("元素")) -> (index of element=w23:i32)  [unwired: 1 in]
  n21 = Search 1D Array(1D array=w9, element=u16 22 ("元素")) -> (index of element=w20:i32)  [unwired: 1 in]
  n22 = for {
    tunnel: w8 -> [w62] mode=indexing
    tunnel: [w57] -> w7 mode=indexing
    tunnel: [w56] -> w6 mode=indexing
    n23 = Unbundle By Name(w62) -> ("String"=w58:string)
    n24 = Concatenate Strings(w58, "固件升级" ("字符串")) -> (w60:string)
    n25 = Obtain Queue(name (unnamed)=w60, element data type=cluster{"selected path":path} {"selected path"=path ""}) -> (queue out=w57:refnum<queue>, error out=w56:errorcluster)  [unwired: 3 in, 1 out]
  }
  n26 = Not Equal?(x=w11, y=-1) -> (x != y?=w5:bool)
  n27 = Not Equal?(x=w14, y=-1) -> (x != y?=w4:bool)
  n28 = Not Equal?(x=w23, y=-1) -> (x != y?=w1:bool)
  n29 = Not Equal?(x=w17, y=-1) -> (x != y?=w3:bool)
  n30 = Not Equal?(x=w20, y=-1) -> (x != y?=w2:bool)
  n31 = case shown="True" w1 {
    frame False {
    }
    frame True {
      n32 = call "反控参数变更.vi"("设置参数"=T9."CODMn") -> ()  [unwired: 11 in]
    }
  }
  n33 = case shown="True" w5 {
    frame False {
    }
    frame True {
      n34 = call "反控参数变更.vi"("设置参数"=T9."氨氮") -> ()  [unwired: 11 in]
    }
  }
  n35 = case shown="True" w4 {
    frame False {
    }
    frame True {
      n36 = call "反控参数变更.vi"("设置参数"=T9."总氮") -> ()  [unwired: 11 in]
    }
  }
  n37 = case shown="True" w3 {
    frame False {
    }
    frame True {
      n38 = call "反控参数变更.vi"("设置参数"=T9."总磷") -> ()  [unwired: 11 in]
    }
  }
  n39 = case shown="True" w2 {
    frame False {
    }
    frame True {
      n40 = call "反控参数变更.vi"("设置参数"=T9."CODCr") -> ()  [unwired: 11 in]
    }
  }
  n41 = case shown="True" w2 {
    tunnel: [_ w69] -> w33
    tunnel: [_ w68] -> w32
    frame False {
    }
    frame True {
      w68 = T10 {"状态告警区"={"系统时间"=timestamp(0 s since 1904-01-01), "工作状态"=0, "测量模式"=enum."待机", "告警代码"=0, "故障代码"=0, "日志代码"=0, "软件版本"=0, "F0"=0.0, "F1"=0.0, "F2"=0.0, "F3"=0.0, "T"=0.0, "H"=0.0, "id"=0, "flowid"=0, "量程"=0, "总磷控温温度1"=0.0, "营养盐控温温度2"=0.0, "ADC"=0.0}, "平台试剂余量百分比"=0.0, "关键参数"={"测量量程"=0.0, "测量精度"=0.0, "测量间隔"=0.0, "消解温度"=0.0, "消解时长"=0.0, "空白校准时间"=timestamp(0 s since 1904-01-01), "曲线截距"=0.0, "曲线斜率"=0.0, "测量检出限"=0.0, "测量信号值"=0.0, "线性相关系数"=0.0, "二次多项式系数"=0.0, "标样校准时间"=timestamp(0 s since 1904-01-01), "稀释倍数"=0.0, "三项式系数"=0.0, "空白标定系数"=0.0, "量程系数"=0.0, "F0/ORPA"=0.0, "F1/ORPB"=0.0, "F2/ORPK"=0.0, "F3"=0.0, "F4"=0.0, "F5"=0.0, "F6"=0.0, "F7"=0.0, "X0/滴定数"=0.0, "量程"=0.0}, "关键参数改变"=FALSE, "校准信息"={"低标液1浓度"=0.0, "低标液1信号值"=0.0, "低标液1启用"=0, "低标液2浓度"=0.0, "低标液2信号值"=0.0, "低标液2启用"=0, "低标液3浓度"=0.0, "低标液3信号值"=0.0, "低标液3启用"=0, "低标液4浓度"=0.0, "低标液4信号值"=0.0, "低标液4启用"=0, "低标液5浓度"=0.0, "低标液5信号值"=0.0, "低标液5启用"=0, "高标液1浓度"=0.0, "高标液1信号值"=0.0, "高标液1启用"=0, "高标液2浓度"=0.0, "高标液2信号值"=0.0, "高标液2启用"=0, "高标液3浓度"=0.0, "高标液3信号值"=0.0, "高标液3启用"=0, "高标液4浓度"=0.0, "高标液4信号值"=0.0, "高标液4启用"=0, "高标液5浓度"=0.0, "高标液5信号值"=0.0, "高标液5启用"=0, "低斜率"=0.0, "低截距"=0.0, "低二次多项式系数"=0.0, "低线性相关系数"=0.0, "高斜率"=0.0, "高截距"=0.0, "高二次多项式系数"=0.0, "高线性相关系数"=0.0}, "校准信息改变"=FALSE, "固件版本号"=""}  # 与CODCr交互全局
      n42 = Obtain Queue(name (unnamed)="CODCr interface Read" ("写入方名称"), element data type=w68) -> (queue out=w69:refnum<queue>)  [unwired: 3 in, 2 out]
    }
  }
  n43 = case shown="True" w1 {
    tunnel: [_ w72] -> w35
    tunnel: [_ w71] -> w34
    frame False {
    }
    frame True {
      w71 = T10 {"状态告警区"={"系统时间"=timestamp(0 s since 1904-01-01), "工作状态"=0, "测量模式"=enum."待机", "告警代码"=0, "故障代码"=0, "日志代码"=0, "软件版本"=0, "F0"=0.0, "F1"=0.0, "F2"=0.0, "F3"=0.0, "T"=0.0, "H"=0.0, "id"=0, "flowid"=0, "量程"=0, "总磷控温温度1"=0.0, "营养盐控温温度2"=0.0, "ADC"=0.0}, "平台试剂余量百分比"=0.0, "关键参数"={"测量量程"=0.0, "测量精度"=0.0, "测量间隔"=0.0, "消解温度"=0.0, "消解时长"=0.0, "空白校准时间"=timestamp(0 s since 1904-01-01), "曲线截距"=0.0, "曲线斜率"=0.0, "测量检出限"=0.0, "测量信号值"=0.0, "线性相关系数"=0.0, "二次多项式系数"=0.0, "标样校准时间"=timestamp(0 s since 1904-01-01), "稀释倍数"=0.0, "三项式系数"=0.0, "空白标定系数"=0.0, "量程系数"=0.0, "F0/ORPA"=0.0, "F1/ORPB"=0.0, "F2/ORPK"=0.0, "F3"=0.0, "F4"=0.0, "F5"=0.0, "F6"=0.0, "F7"=0.0, "X0/滴定数"=0.0, "量程"=0.0}, "关键参数改变"=FALSE, "校准信息"={"低标液1浓度"=0.0, "低标液1信号值"=0.0, "低标液1启用"=0, "低标液2浓度"=0.0, "低标液2信号值"=0.0, "低标液2启用"=0, "低标液3浓度"=0.0, "低标液3信号值"=0.0, "低标液3启用"=0, "低标液4浓度"=0.0, "低标液4信号值"=0.0, "低标液4启用"=0, "低标液5浓度"=0.0, "低标液5信号值"=0.0, "低标液5启用"=0, "高标液1浓度"=0.0, "高标液1信号值"=0.0, "高标液1启用"=0, "高标液2浓度"=0.0, "高标液2信号值"=0.0, "高标液2启用"=0, "高标液3浓度"=0.0, "高标液3信号值"=0.0, "高标液3启用"=0, "高标液4浓度"=0.0, "高标液4信号值"=0.0, "高标液4启用"=0, "高标液5浓度"=0.0, "高标液5信号值"=0.0, "高标液5启用"=0, "低斜率"=0.0, "低截距"=0.0, "低二次多项式系数"=0.0, "低线性相关系数"=0.0, "高斜率"=0.0, "高截距"=0.0, "高二次多项式系数"=0.0, "高线性相关系数"=0.0}, "校准信息改变"=FALSE, "固件版本号"=""}  # 与CODMn交互全局
      n44 = Obtain Queue(name (unnamed)="CODMn interface Read" ("写入方名称"), element data type=w71) -> (queue out=w72:refnum<queue>)  [unwired: 3 in, 2 out]
    }
  }
  n45 = case shown="True" w5 {
    tunnel: [_ w75] -> w27
    tunnel: [_ w74] -> w26
    frame False {
    }
    frame True {
      w74 = T11 {"状态告警区"={"系统时间"=timestamp(0 s since 1904-01-01), "工作状态"=0, "测量模式"=enum."待机", "告警代码"=0, "故障代码"=0, "日志代码"=0, "软件版本"=0, "F0"=0.0, "F1"=0.0, "F2"=0.0, "F3"=0.0, "T"=0.0, "H"=0.0, "id"=0, "flowid"=0, "量程"=0, "总磷控温温度1"=0.0, "营养盐控温温度2"=0.0, "ADC"=0.0}, "平台试剂余量百分比"=0.0, "关键参数"={"测量量程"=0.0, "测量精度"=0.0, "测量间隔"=0.0, "消解温度"=0.0, "消解时长"=0.0, "空白校准时间"=timestamp(0 s since 1904-01-01), "曲线截距"=0.0, "曲线斜率"=0.0, "测量检出限"=0.0, "测量信号值"=0.0, "线性相关系数"=0.0, "二次多项式系数"=0.0, "标样校准时间"=timestamp(0 s since 1904-01-01), "稀释倍数"=0.0, "三项式系数"=0.0, "空白标定系数"=0.0, "量程系数"=0.0, "F0/ORPA"=0.0, "F1/ORPB"=0.0, "F2/ORPK"=0.0, "F3"=0.0, "F4"=0.0, "F5"=0.0, "F6"=0.0, "F7"=0.0, "X0/滴定数"=0.0, "量程"=0.0}, "关键参数改变"=FALSE, "校准信息"={"低标液1浓度"=0.0, "低标液1信号值"=0.0, "低标液1启用"=0, "低标液2浓度"=0.0, "低标液2信号值"=0.0, "低标液2启用"=0, "低标液3浓度"=0.0, "低标液3信号值"=0.0, "低标液3启用"=0, "低标液4浓度"=0.0, "低标液4信号值"=0.0, "低标液4启用"=0, "低标液5浓度"=0.0, "低标液5信号值"=0.0, "低标液5启用"=0, "高标液1浓度"=0.0, "高标液1信号值"=0.0, "高标液1启用"=0, "高标液2浓度"=0.0, "高标液2信号值"=0.0, "高标液2启用"=0, "高标液3浓度"=0.0, "高标液3信号值"=0.0, "高标液3启用"=0, "高标液4浓度"=0.0, "高标液4信号值"=0.0, "高标液4启用"=0, "高标液5浓度"=0.0, "高标液5信号值"=0.0, "高标液5启用"=0, "低斜率"=0.0, "低截距"=0.0, "低二次多项式系数"=0.0, "低线性相关系数"=0.0, "高斜率"=0.0, "高截距"=0.0, "高二次多项式系数"=0.0, "高线性相关系数"=0.0}, "校准信息改变"=FALSE, "固件版本号"=""}  # 与氨氮交互全局
      n46 = Obtain Queue(name (unnamed)="氨氮 interface Read" ("写入方名称"), element data type=w74) -> (queue out=w75:refnum<queue>)  [unwired: 3 in, 2 out]
    }
  }
  n47 = case shown="True" w4 {
    tunnel: [_ w78] -> w29
    tunnel: [_ w77] -> w28
    frame False {
    }
    frame True {
      w77 = T12 {"状态告警区"={"系统时间"=timestamp(0 s since 1904-01-01), "工作状态"=0, "测量模式"=enum."待机", "告警代码"=0, "故障代码"=0, "日志代码"=0, "软件版本"=0, "F0"=0.0, "F1"=0.0, "F2"=0.0, "F3"=0.0, "T"=0.0, "H"=0.0, "id"=0, "flowid"=0, "量程"=0, "总磷控温温度1"=0.0, "营养盐控温温度2"=0.0, "ADC"=0.0}, "平台试剂余量百分比"=0.0, "关键参数"={"测量量程"=0.0, "测量精度"=0.0, "测量间隔"=0.0, "消解温度"=0.0, "消解时长"=0.0, "空白校准时间"=timestamp(0 s since 1904-01-01), "曲线截距"=0.0, "曲线斜率"=0.0, "测量检出限"=0.0, "测量信号值"=0.0, "线性相关系数"=0.0, "二次多项式系数"=0.0, "标样校准时间"=timestamp(0 s since 1904-01-01), "稀释倍数"=0.0, "三项式系数"=0.0, "空白标定系数"=0.0, "量程系数"=0.0, "F0/ORPA"=0.0, "F1/ORPB"=0.0, "F2/ORPK"=0.0, "F3"=0.0, "F4"=0.0, "F5"=0.0, "F6"=0.0, "F7"=0.0, "X0/滴定数"=0.0, "量程"=0.0}, "关键参数改变"=FALSE, "校准信息"={"低标液1浓度"=0.0, "低标液1信号值"=0.0, "低标液1启用"=0, "低标液2浓度"=0.0, "低标液2信号值"=0.0, "低标液2启用"=0, "低标液3浓度"=0.0, "低标液3信号值"=0.0, "低标液3启用"=0, "低标液4浓度"=0.0, "低标液4信号值"=0.0, "低标液4启用"=0, "低标液5浓度"=0.0, "低标液5信号值"=0.0, "低标液5启用"=0, "高标液1浓度"=0.0, "高标液1信号值"=0.0, "高标液1启用"=0, "高标液2浓度"=0.0, "高标液2信号值"=0.0, "高标液2启用"=0, "高标液3浓度"=0.0, "高标液3信号值"=0.0, "高标液3启用"=0, "高标液4浓度"=0.0, "高标液4信号值"=0.0, "高标液4启用"=0, "高标液5浓度"=0.0, "高标液5信号值"=0.0, "高标液5启用"=0, "低斜率"=0.0, "低截距"=0.0, "低二次多项式系数"=0.0, "低线性相关系数"=0.0, "高斜率"=0.0, "高截距"=0.0, "高二次多项式系数"=0.0, "高线性相关系数"=0.0}, "校准信息改变"=FALSE, "固件版本号"=""}  # 与总氮交互全局
      n48 = Obtain Queue(name (unnamed)="总氮 interface Read" ("写入方名称"), element data type=w77) -> (queue out=w78:refnum<queue>)  [unwired: 3 in, 2 out]
    }
  }
  n49 = case shown="True" w3 {
    tunnel: [_ w81] -> w31
    tunnel: [_ w80] -> w30
    frame False {
    }
    frame True {
      w80 = T13 {"状态告警区"={"系统时间"=timestamp(0 s since 1904-01-01), "工作状态"=0, "测量模式"=enum."待机", "告警代码"=0, "故障代码"=0, "日志代码"=0, "软件版本"=0, "F0"=0.0, "F1"=0.0, "F2"=0.0, "F3"=0.0, "T"=0.0, "H"=0.0, "id"=0, "flowid"=0, "量程"=0, "总磷控温温度1"=0.0, "营养盐控温温度2"=0.0, "ADC"=0.0}, "平台试剂余量百分比"=0.0, "关键参数"={"测量量程"=0.0, "测量精度"=0.0, "测量间隔"=0.0, "消解温度"=0.0, "消解时长"=0.0, "空白校准时间"=timestamp(0 s since 1904-01-01), "曲线截距"=0.0, "曲线斜率"=0.0, "测量检出限"=0.0, "测量信号值"=0.0, "线性相关系数"=0.0, "二次多项式系数"=0.0, "标样校准时间"=timestamp(0 s since 1904-01-01), "稀释倍数"=0.0, "三项式系数"=0.0, "空白标定系数"=0.0, "量程系数"=0.0, "F0/ORPA"=0.0, "F1/ORPB"=0.0, "F2/ORPK"=0.0, "F3"=0.0, "F4"=0.0, "F5"=0.0, "F6"=0.0, "F7"=0.0, "X0/滴定数"=0.0, "量程"=0.0}, "关键参数改变"=FALSE, "校准信息"={"低标液1浓度"=0.0, "低标液1信号值"=0.0, "低标液1启用"=0, "低标液2浓度"=0.0, "低标液2信号值"=0.0, "低标液2启用"=0, "低标液3浓度"=0.0, "低标液3信号值"=0.0, "低标液3启用"=0, "低标液4浓度"=0.0, "低标液4信号值"=0.0, "低标液4启用"=0, "低标液5浓度"=0.0, "低标液5信号值"=0.0, "低标液5启用"=0, "高标液1浓度"=0.0, "高标液1信号值"=0.0, "高标液1启用"=0, "高标液2浓度"=0.0, "高标液2信号值"=0.0, "高标液2启用"=0, "高标液3浓度"=0.0, "高标液3信号值"=0.0, "高标液3启用"=0, "高标液4浓度"=0.0, "高标液4信号值"=0.0, "高标液4启用"=0, "高标液5浓度"=0.0, "高标液5信号值"=0.0, "高标液5启用"=0, "低斜率"=0.0, "低截距"=0.0, "低二次多项式系数"=0.0, "低线性相关系数"=0.0, "高斜率"=0.0, "高截距"=0.0, "高二次多项式系数"=0.0, "高线性相关系数"=0.0}, "校准信息改变"=FALSE, "固件版本号"=""}  # 与总磷交互全局
      n50 = Obtain Queue(name (unnamed)="总磷 interface Read" ("写入方名称"), element data type=w80) -> (queue out=w81:refnum<queue>)  [unwired: 3 in, 2 out]
    }
  }
  n51 = Obtain Queue(name (unnamed)=w36, element data type=w41) -> (queue out=w37:refnum<queue>, error out=w40:errorcluster)  [unwired: 3 in, 1 out]
  n52 = while {
    tunnel: w7 -> [w87]
    tunnel: w6 -> [w86]
    tunnel: [w85] -> _
    tunnel: [w84] -> _
    stop <- FALSE stop-if-true
    n53 = for {
      tunnel: w87 -> [w94] mode=indexing
      tunnel: w86 -> [w93] mode=indexing
      tunnel: [w92] -> w85
      tunnel: [w91] -> w84
      n54 = Dequeue Element(queue=w94, timeout in ms (-1)=1000 ("超时毫秒(-1)"), error in (no error)=w93) -> (queue out=w92:refnum<queue>, element=w90:cluster{"selected path":path}, timed out?=w88:bool, error out=w91:errorcluster)
      n55 = case shown="False" w88 {
        tunnel: w90 -> [w103 _]
        frame False {
          n56 = Unbundle By Name(w103) -> ("selected path"=w102:path)
          n57 = call "固件升级（包含参数恢复）.vi"("路径对话框"=FALSE, "selected path"=w102) -> ("结果字符串"=w96:string)  [unwired: 9 in]
          n58 = global read "VAR总磷总氮全局变量.vi" "模块名称"() -> (w98:string)
          n59 = Concatenate Strings("平台反控固件升级" ("日志信息"), w96) -> (w95:string)
          n60 = Get Date/Time In Seconds() -> (seconds since 1Jan1904=w99:timestamp)
          n61 = Bundle By Name(cluster=T14 {"时间"=timestamp(0 s since 1904-01-01), "参数"="", "日志信息"="", "流程参数"=""} ("data in"), "时间"=w99, "参数"=w98, "日志信息"=w95) -> (w100:T14)
          n62 = call "总磷总氮操作日志.vi"("data in"=w100) -> ()  [unwired: 10 in, 1 out]
        }
        frame True {
        }
      }
    }
  }
  n63 = Generate Occurrence() -> (w38:refnum<k4>)
  n64 = while {
    tunnel: w37 -> [w107]
    tunnel: w38 -> [w105]
    stop <- w106 stop-if-true
    n65 = event shown="[3] \"启动\": Value Change" {
      selector: _ -> [_ _ _ _ _ _ _ _]
      dyn-events: _ -> [_ _ _ _ _ _ _ _]
      timeout: _ -> [_ _ _ _ _ _ _ _]
      tunnel: w107 -> [_ _ _ w139 w149 w155 w160 w165]
      tunnel: [_ _ _ _ "停止" _ _ _] -> w106
      tunnel: w105 -> [_ _ _ _ w146 _ _ _]
      event Timeout {
        n66 = event-data() -> ()  [unwired: 1 in, 3 out]
      }
      event "启用模块": Value Change {
        n67 = event-data() -> ("NewVal"=w108:bool)  [unwired: 1 in, 5 out]
        n68 = call <vilib>:"Application Directory.vi"() -> ("Application Directory"=w110:path)
        n69 = Build Path(base path=w110, name or relative path="data\\set.ini" ("名称或相对路径")) -> (appended path=w111:path)
        n70 = call <vilib>:"Open Config Data.vi"("configuration file path"=w111) -> ("error out"=w117:errorcluster, "refnum"=w116:T15)  [unwired: 8 in, 1 out]
        n71 = call-poly <vilib>:"Write Key.vi"("section"="总磷总氮", "error in (no error)"=w117, "value"=w108, "key"="模块启用", "refnum"=w116) -> ("error out"=w113:errorcluster, "refnum out"=w109:T15)  [unwired: 4 in, 1 out]
        n72 = call <vilib>:"Close Config Data.vi"("error in (no error)"=w113, "refnum"=w109) -> ()  [unwired: 8 in, 2 out]
      }
      event "VISA Resource": Value Change {
        n73 = event-data() -> ()  [unwired: 1 in, 6 out]
        n74 = call <vilib>:"Application Directory.vi"() -> ("Application Directory"=w120:path)
        n75 = Build Path(base path=w120, name or relative path="data\\set.ini" ("名称或相对路径")) -> (appended path=w121:path)
        n76 = call <vilib>:"Open Config Data.vi"("configuration file path"=w121) -> ("error out"=w127:errorcluster, "refnum"=w126:T15)  [unwired: 8 in, 1 out]
        n77 = call-poly <vilib>:"Write Key.vi"("section"="总磷总氮", "error in (no error)"=w127, "value"="VISA Resource", "key"="串口", "refnum"=w126) -> ("error out"=w123:errorcluster, "refnum out"=w119:T15)  [unwired: 4 in, 1 out]
        n78 = call <vilib>:"Close Config Data.vi"("error in (no error)"=w123, "refnum"=w119) -> ()  [unwired: 8 in, 2 out]
      }
      event "启动": Value Change {
        n79 = event-data() -> ()  [unwired: 1 in, 6 out]
        n80 = global read "总磷总氮断电保存全局变量.vi" "协议"() -> (w128:u16)
        n81 = case shown="2" w128 {
          tunnel: [w140 w142] -> w132
          tunnel: "控制命令" -> [w140 w141]
          frame 2 {
          }
          frame 1, Default {
            n82 = Swap Bytes(anything=w141) -> (byte swapped=w142:u16)
          }
        }
        n83 = case shown="Default" "控制命令" {
          tunnel: "控制命令参数" -> [w144 w145]
          tunnel: [w143 w145] -> w129
          frame Default {
            n84 = call "HexToWord.vi"("数组"=w144) -> ("WORD"=w143:u16[])  [unwired: 10 in]
          }
          frame 13 {
          }
        }
        n85 = call "控制命令区.vi"("控制命令参数"=w129, "控制命令"=w132) -> ("控制命令"=w135:u16[])  [unwired: 9 in]
        n86 = local read "站号"() -> (w134:u16)
        n87 = Bundle("站号"=w134, "控制命令"=w135) -> (w133:cluster{"站号":u16, "控制命令":u16[]})  [unwired: 1 in]
        n88 = Bundle By Name(cluster=cluster{"命令":string, "data":variant} {"命令"="", "data"=variant} ("元素"), "命令"="启动", "data"=w133) -> (w137:cluster{"命令":string, "data":variant})
        n89 = Enqueue Element(queue=w139, element=w137) -> ()  [unwired: 2 in, 3 out]
      }
      event "停止": Value Change {
        n90 = event-data() -> ()  [unwired: 1 in, 6 out]
        n91 = Set Occurrence(w146) -> ()
        n92 = Flush Queue(queue=w149) -> (queue out=w148:refnum<queue>)  [unwired: 1 in, 2 out]
        n93 = Enqueue Element(queue=w148, element=cluster{"命令":string, "data":variant} {"命令"="shutdown", "data"=variant} ("元素")) -> ()  [unwired: 2 in, 3 out]
      }
      event "读测量数据区": Value Change {
        n94 = event-data() -> ()  [unwired: 1 in, 6 out]
        n95 = Bundle By Name(cluster=cluster{"命令":string, "data":variant} {"命令"="", "data"=variant} ("元素"), "命令"="读测量数据区", "data"="站号") -> (w153:cluster{"命令":string, "data":variant})
        n96 = Enqueue Element(queue=w155, element=w153) -> ()  [unwired: 2 in, 3 out]
      }
      event "读状态告警区": Value Change {
        n97 = event-data() -> ()  [unwired: 1 in, 6 out]
        n98 = local read "站号"() -> (w156:u16)
        n99 = Bundle By Name(cluster=cluster{"命令":string, "data":variant} {"命令"="", "data"=variant} ("元素"), "命令"="读状态告警区", "data"=w156) -> (w158:cluster{"命令":string, "data":variant})
        n100 = Enqueue Element(queue=w160, element=w158) -> ()  [unwired: 2 in, 3 out]
      }
      event "读关键参数区": Value Change {
        n101 = event-data() -> ()  [unwired: 1 in, 6 out]
        n102 = local read "站号"() -> (w161:u16)
        n103 = Bundle By Name(cluster=cluster{"命令":string, "data":variant} {"命令"="", "data"=variant} ("元素"), "命令"="读关键参数区", "data"=w161) -> (w163:cluster{"命令":string, "data":variant})
        n104 = Enqueue Element(queue=w165, element=w163) -> ()  [unwired: 2 in, 3 out]
      }
    }
  }
  n105 = while {
    tunnel: w38 -> [w176]
    tunnel: w37 -> [w172]
    stop <- w173 stop-if-true
    n106 = global read "总磷总氮断电保存全局变量.vi" "MB通信方式选择"() -> (w171:enum16{"串口", "TCP"})
    n107 = Wait on Occurrence(2:w176, 3:10000 ("毫秒超时(-1)")) -> (0:w174:bool)  [unwired: 1 in]
    n108 = Not(x=w174) -> (.not. x?=w173:bool)
    n109 = case shown="\"TCP\"" w171 {
      tunnel: [_ w177] -> w168
      frame "串口", Default {
      }
      frame "TCP" {
        n110 = global read "VAR总磷总氮全局变量.vi" "MB session in"() -> (w179:refnum<class "MB_Master.lvclass">)
        n111 = property class="MB_Master"(reference=w179) -> ("Properties:Session Valid"=w178:bool)  [unwired: 1 in, 2 out]
        n112 = Not(x=w178) -> (.not. x?=w177:bool)
      }
    }
    n113 = First Call?() -> (First Call?: T/F=w170:bool)
    n114 = Or(x=w168, y=w170) -> (x .or. y?=w169:bool)
    n115 = local read "启用"() -> (w166:bool)
    n116 = And(x=w166, y=w169) -> (x .and. y?=w167:bool)
    n117 = case shown="True" w167 {
      tunnel: w172 -> [_ w182]
      frame False {
      }
      frame True {
        n118 = Flush Queue(queue=w182) -> (queue out=w180:refnum<queue>)  [unwired: 1 in, 2 out]
        n119 = Enqueue Element(queue=w180, element=cluster{"命令":string, "data":variant} {"命令"="启用模块", "data"=variant} ("元素")) -> ()  [unwired: 2 in, 3 out]
        n120 = property on="VISA Resource" class="VISAName"("DisabledEnum"=T16."Disabled and Grayed Out" ("禁用")) -> ()  [unwired: 2 in, 2 out]
      }
    }
  }
  n121 = while {
    tunnel: w37 -> [w200]
    tunnel: w40 -> [w199]
    shift-right: [w186] -> _
    shift-left: _ -> [w197]
    tunnel: errorcluster {"status"=FALSE, "code"=0, "source"=""} ("error out") -> [w196]
    tunnel: [w192] -> _
    stop <- w198 stop-if-true
    n122 = Dequeue Element(queue=w200, error in (no error)=w199) -> (queue out=w193:refnum<queue>, element=w194:cluster{"命令":string, "data":variant})  [unwired: 1 in, 2 out]
    n123 = Unbundle By Name(w194) -> ("命令"=w195:string, "data"=w190:variant)
    n124 = case shown="\"读测量数据区\"" w195 {
      tunnel: w190 -> [_ _ _ w237 w248 w265 w273 w398 w458 _]
      tunnel: w193 -> [_ _ _ _ _ _ w274 _ _ w471]
      tunnel: [_ _ _ _ _ _ _ _ _ TRUE] -> w198
      tunnel: [w203 w206 w224 w240 w251 w267 w295 w406 w465 w467] -> w186
      tunnel: [w204 w205 w225 w239 w250 w266 w296 w397 w466 w468] -> w192
      tunnel: w197 -> [w203 _ w224 w236 w247 w264 w291 w401 w461 w467]
      tunnel: w196 -> [w204 _ w226 w233 w244 w261 w289 w402 w462 w469]
      tunnel: [_ _ _ w228 w241 w255 w270 w379 w452 _] -> w184
      frame Default {
      }
      frame "启用模块" {
        n125 = global read "总磷总氮断电保存全局变量.vi" "MB通信方式选择"() -> (w207:enum16{"串口", "TCP"})
        n126 = case shown="\"串口\", Default" w207 {
          tunnel: [w215 w220] -> w205
          tunnel: [w212 w219] -> w206
          frame "串口", Default {
            n127 = global read "总磷总氮断电保存全局变量.vi" "波特率"() -> (w210:u32)
            n128 = Bundle By Name(cluster=T17 {"baud rate (bps)"=115200, "stop bits"=10, "parity"=0, "flow control"=0, "timeout"=1000, "retries"=1} ("Serial Config"), "baud rate (bps)"=w210) -> (w209:T17)
            n129 = global read "总磷总氮断电保存全局变量.vi" "VISA Resource"() -> (w213:refnum<visa-resource-name>)
            n130 = call <vilib>:"Open Serial Session.vi"("Mode (RTU)"=enum16{"RTU", "ASCII"}."RTU", "Slave ID"=u8 1, "Serial Config"=w209, "VISA Resource"=w213) -> ("Error out"=w215:errorcluster, "MB_Serial session"=w212:refnum<class "MB_Master_Serial.lvclass">)  [unwired: 6 in]
          }
          frame "TCP" {
            n131 = global read "总磷总氮断电保存全局变量.vi" "PORT"() -> (w218:string)
            n132 = Decimal String To Number(string=w218) -> (number=w221:i32)  [unwired: 2 in, 1 out]
            n133 = global read "总磷总氮断电保存全局变量.vi" "IP"() -> (w217:string)
            n134 = call <vilib>:"Open TCP Session.vi"("Port (502)"=w221, "IP Address"=w217) -> ("error out"=w220:errorcluster, "MB_TCP session"=w219:refnum<class "MB_Master_TCP.lvclass">)  [unwired: 8 in]
          }
        }
        "启用" <- TRUE
      }
      frame "停用模块" {
        n135 = call-dynamic "Close Session.vi"("error in (no error)"=w226, "MB session in"=w224) -> ("error out"=w222:errorcluster)  [unwired: 9 in]
        n136 = local write "启用"(FALSE ("启用")) -> ()
        n137 = call <vilib>:"Clear Errors.vi"("error in (no error)"=w222) -> ("error out"=w225:errorcluster)  [unwired: 5 in, 1 out]
      }
      frame "启动" {
        n138 = Variant To Data(type=cluster{"站号":u16, "控制命令":u16[]} {"站号"=0, "控制命令"=[]} ("输出簇"), Variant=w237) -> (data=w231:cluster{"站号":u16, "控制命令":u16[]})  [unwired: 1 in, 1 out]
        n139 = Unbundle By Name(w231) -> ("站号"=w228:u16, "控制命令"=w229:u16[])
        n140 = property class="MB_Master"(reference=w236, error in=w233, "Properties:Slave ID"=w228) -> (reference out=w235:refnum<class "MB_Master.lvclass">, error out=w234:errorcluster)
        n141 = Index Array(array=w229) -> (element=w230:u16)  [unwired: 1 in]
        n142 = Swap Bytes(anything=w230) -> (byte swapped=w227:u16)
        n143 = global write "VAR总磷总氮全局变量.vi" "控制命令"(w227) -> ()
        n144 = call <vilib>:"Write Multiple Registers.vi"("error in (no error)"=w234, "values"=w229, "starting address"=u16 4608, "MB session in"=w235) -> ("error out"=w239:errorcluster, "MB session out"=w240:refnum<class "MB_Master.lvclass">)  [unwired: 6 in]
      }
      frame "盲样测试" {
        n145 = Variant To Data(type=u8 0, Variant=w248) -> (data=w241:u8)  [unwired: 1 in, 1 out]
        n146 = property class="MB_Master"(reference=w247, error in=w244, "Properties:Slave ID"=w241) -> (reference out=w246:refnum<class "MB_Master.lvclass">, error out=w245:errorcluster)
        n147 = case shown="Default" w241 {
          tunnel: [u16[] [] ("values") u16[] [33539, 0] ("values") u16[] [23555, 0] ("values")] -> w243
          frame Default {
          }
          frame 1 {
            # "总磷盲样测试命令"
          }
          frame 3 {
            # "氨氮盲样测试"
          }
        }
        n148 = call <vilib>:"Write Multiple Registers.vi"("error in (no error)"=w245, "values"=w243, "starting address"=u16 24592, "MB session in"=w246) -> ("error out"=w250:errorcluster, "MB session out"=w251:refnum<class "MB_Master.lvclass">)  [unwired: 6 in]
      }
      frame "debug" {
        n149 = Variant To Data(type=cluster{"站号":u16, "控制命令":u16[]} {"站号"=0, "控制命令"=[]} ("输出簇"), Variant=w265) -> (data=w259:cluster{"站号":u16, "控制命令":u16[]})  [unwired: 1 in, 1 out]
        n150 = Unbundle By Name(w259) -> ("站号"=w255:u16, "控制命令"=w257:u16[])
        n151 = property class="MB_Master"(reference=w264, error in=w261, "Properties:Slave ID"=w255) -> (reference out=w263:refnum<class "MB_Master.lvclass">, error out=w262:errorcluster)
        n152 = Index Array(array=w257) -> (element=w258:u16)  [unwired: 1 in]
        n153 = global write "VAR总磷总氮全局变量.vi" "控制命令"(w258) -> ()
        n154 = call <vilib>:"Write Multiple Registers.vi"("error in (no error)"=w262, "values"=w257, "starting address"=u16 24594, "MB session in"=w263) -> ("error out"=w266:errorcluster, "MB session out"=w267:refnum<class "MB_Master.lvclass">)  [unwired: 6 in]
      }
      frame "读测量数据区" {
        n155 = global read "model config var.vi" "启动队列名称"() -> (w271:cluster{"String":string, "Value":u16}[])
        n156 = Bundle("命令"="读关键参数区", "data"=w273) -> (w275:cluster{"命令":string, "data":variant})  [unwired: 1 in]
        n157 = Variant To Data(type=u8 1 ("Slave ID"), Variant=w273) -> (data=w270:u8)  [unwired: 1 in, 1 out]
        n158 = property class="MB_Master"(reference=w291, error in=w289, "Properties:Slave ID"=w270) -> (reference out=w290:refnum<class "MB_Master.lvclass">, error out=w288:errorcluster)
        n159 = Enqueue Element(queue=w274, element=w275) -> ()  [unwired: 2 in, 3 out]
        n160 = Index Array(array=w271) -> (element=w272:cluster{"String":string, "Value":u16})  [unwired: 1 in]
        n161 = Unbundle By Name(w272) -> ("Value"=w268:u16)
        n162 = global read "VAR总磷总氮全局变量.vi" "测量数据区数组"() -> (w285:T8)
        n163 = Not Equal?(x=w268, y=w270) -> (x != y?=w269:bool)
        n164 = call "id参数转换.vi"("id"=w268) -> ("数组资源索引"=w280:i32)  [unwired: 9 in, 1 out]
        n165 = call <vilib>:"Read Holding Registers.vi"("error in (no error)"=w288, "quantity"=u16 107, "starting address"=u16 4096, "MB session in"=w290) -> ("error out"=w296:errorcluster, "Registers"=w287:u16[], "MB session out"=w295:refnum<class "MB_Master.lvclass">)  [unwired: 5 in]
        n166 = call "id参数转换.vi"("id"=w270) -> ("数组资源索引"=w281:i32)  [unwired: 9 in, 1 out]
        n167 = Index Array(array=w285, index #1=w281, index #2=w280) -> (element #1=w286:T5, element #2=w282:T5)
        n168 = call "测量数据区.vi"("数组"=w287) -> ("测量数据区"=w277:T5)  [unwired: 10 in]
        "测量数据区" <- w277
        n169 = global write "VAR总磷总氮全局变量.vi" "测量数据区"(w277) -> ()
        n170 = global read "工况数据接口全局.vi" "data"() -> (w279:T18)
        n171 = case shown="0, Default" w270 {
          selector: w270 -> [w302 _ _ _ _]
          tunnel: w277 -> [w298 w343 w353 w366 w373]
          tunnel: w287 -> [_ w347 w365 w372 w378]
          tunnel: w286 -> [w300 w345 _ _ _]
          tunnel: [w297 w346 w353 w366 w373] -> w284
          tunnel: w282 -> [w299 w335 _ _ _]
          tunnel: w279 -> [w303 w344 w364 w371 w377]
          tunnel: [w303 w337 w354 w367 w376] -> w278
          tunnel: w269 -> [w301 w336 _ _ _]
          frame 0, Default {
            n172 = case shown="4" w302 {
              tunnel: w301 -> [_ w309 w319 w329]
              tunnel: w300 -> [_ w308 w318 w328]
              tunnel: w299 -> [_ w307 w317 w327]
              tunnel: w298 -> [w304 w306 w316 w326]
              tunnel: [w304 w305 w315 w325] -> w297
              frame 0, Default {
              }
              frame 4 {
                n173 = case shown="False" w309 {
                  tunnel: w308 -> [_ w314]
                  tunnel: w307 -> [_ w313]
                  tunnel: w306 -> [w310 w312]
                  tunnel: [w310 w311] -> w305
                  frame False {
                  }
                  frame True {
                    n174 = call "数据时间对齐.vi"("待对齐时间"=w312, "对齐参考时间"=w313, "已对齐时间输入"=w314) -> ("已对齐时间输出"=w311:T5)  [unwired: 8 in]
                  }
                }
              }
              frame 5 {
                n175 = case shown="False" w319 {
                  tunnel: w318 -> [_ w324]
                  tunnel: w317 -> [_ w323]
                  tunnel: w316 -> [w320 w322]
                  tunnel: [w320 w321] -> w315
                  frame False {
                  }
                  frame True {
                    n176 = call "数据时间对齐.vi"("待对齐时间"=w322, "对齐参考时间"=w323, "已对齐时间输入"=w324) -> ("已对齐时间输出"=w321:T5)  [unwired: 8 in]
                  }
                }
              }
              frame 6 {
                n177 = case shown="False" w329 {
                  tunnel: w328 -> [_ w334]
                  tunnel: w327 -> [_ w333]
                  tunnel: w326 -> [w330 w332]
                  tunnel: [w330 w331] -> w325
                  frame False {
                  }
                  frame True {
                    n178 = call "数据时间对齐.vi"("待对齐时间"=w332, "对齐参考时间"=w333, "已对齐时间输入"=w334) -> ("已对齐时间输出"=w331:T5)  [unwired: 8 in]
                  }
                }
              }
            }
          }
          frame 1 {
            n179 = Unbundle By Name(w343) -> ("F0"=w342:sgl, "F1"=w341:sgl, "F2"=w340:sgl, "F3"=w339:sgl, "X值"=w338:sgl)
            n180 = case shown="True" w336 {
              tunnel: [w348 w352] -> w346
              tunnel: w345 -> [_ w351]
              tunnel: w335 -> [_ w350]
              tunnel: w343 -> [w348 w349]
              frame False {
              }
              frame True {
                # "启动总磷总氮时间自动对齐"
                n181 = call "数据时间对齐.vi"("待对齐时间"=w349, "对齐参考时间"=w350, "已对齐时间输入"=w351) -> ("已对齐时间输出"=w352:T5)  [unwired: 8 in]
              }
            }
            n182 = Bundle By Name(cluster=w344, "data.TP.TP.F0"=w342, "data.TP.TP.F1"=w341, "data.TP.TP.F2"=w340, "data.TP.TP.F3"=w339, "data.TP.TP.X0"=w338) -> (w337:T18)
            "总磷测量数据区" <- w347
          }
          frame 2 {
            n183 = Unbundle By Name(w353) -> ("F0"=w363:sgl, "F1"=w362:sgl, "F2"=w361:sgl, "F3"=w360:sgl, "F4"=w359:sgl, "F5"=w358:sgl, "F6"=w357:sgl, "F7"=w356:sgl, "X值"=w355:sgl)
            n184 = Bundle By Name(cluster=w364, "data.TN.TN.F0"=w363, "data.TN.TN.F1"=w362, "data.TN.TN.F2"=w361, "data.TN.TN.F3"=w360, "data.TN.TN.F4"=w359, "data.TN.TN.F5"=w358, "data.TN.TN.F6"=w357, "data.TN.TN.F7"=w356, "data.TN.TN.X0"=w355) -> (w354:T18)
            "总氮测量数据区" <- w365
          }
          frame 3 {
            n185 = Unbundle By Name(w366) -> ("F0"=w370:sgl, "F1"=w369:sgl, "X值"=w368:sgl)
            n186 = Bundle By Name(cluster=w371, "data.NH3.NH3.F0"=w370, "data.NH3.NH3.F1"=w369, "data.NH3.NH3.X0"=w368) -> (w367:T18)
            "氨氮测量数据区" <- w372
          }
          frame 22 {
            n187 = Unbundle By Name(w373) -> ("F0"=w375:sgl, "F1"=w374:sgl)
            n188 = Bundle By Name(cluster=w377, "data.CODCr.CODCr.F0"=w375, "data.CODCr.CODCr.F1"=w374) -> (w376:T18)
            "COD测量数据区" <- w378
          }
        }
        n189 = global write "工况数据接口全局.vi" "data"(w278) -> ()
        n190 = Replace Array Subset(array=w285, new element=w284, index=w281) -> (w283:T8)
        n191 = global write "VAR总磷总氮全局变量.vi" "测量数据区数组"(w283) -> ()
      }
      frame "读状态告警区" {
        n192 = Variant To Data(type=u8 1 ("Slave ID"), Variant=w398) -> (data=w379:u8)  [unwired: 1 in, 1 out]
        n193 = property class="MB_Master"(reference=w401, error in=w402, "Properties:Slave ID"=w379) -> (reference out=w400:refnum<class "MB_Master.lvclass">, error out=w399:errorcluster)
        n194 = call "id参数转换.vi"("id"=w379) -> ("数组资源索引"=w392:i32)  [unwired: 9 in, 1 out]
        n195 = call <vilib>:"Read Holding Registers.vi"("error in (no error)"=w399, "quantity"=u16 44, "starting address"=u16 4224, "MB session in"=w400) -> ("error out"=w397:errorcluster, "Registers"=w395:u16[], "MB session out"=w406:refnum<class "MB_Master.lvclass">)  [unwired: 5 in]
        n196 = global read "VAR总磷总氮全局变量.vi" "状态告警区数组"() -> (w394:T7)
        n197 = call "状态告警区.vi"("数组"=w395) -> ("状态告警区 2"=w380:T19, "状态告警区"=w381:T4)  [unwired: 9 in]
        "状态告警区" <- w380
        n198 = Unbundle By Name(w381) -> ("日志代码"=w382:u16, "告警代码"=w388:u16, "故障代码"=w386:u16)
        n199 = global write "VAR总磷总氮全局变量.vi" "状态告警区"(w380) -> ()
        n200 = Unbundle By Name(w381) -> ("id"=w396:u16)
        n201 = Replace Array Subset(array=w394, new element=w381, index=w392) -> (w393:T7)
        n202 = global write "VAR总磷总氮全局变量.vi" "状态告警区数组"(w393) -> ()
        n203 = feedback-in #1(w388) -> ()
        n204 = feedback #1() -> (w389:u16)  [unwired: 1 in]
        n205 = feedback #2() -> (w387:u16)  [unwired: 1 in]
        n206 = feedback-in #2(w386) -> ()
        n207 = Not Equal?(x=w389, y=w388) -> (x != y?=w385:bool)
        n208 = Not Equal?(x=w387, y=w386) -> (x != y?=w384:bool)
        n209 = Or(x=w385, y=w384) -> (x .or. y?=w383:bool)
        n210 = global read "工况数据接口全局.vi" "data"() -> (w391:T18)
        n211 = case shown="2, 76" w396 {
          tunnel: w381 -> [_ w419 w432 w442 w448]
          tunnel: w395 -> [_ w420 w433 w443 w450]
          tunnel: w391 -> [w407 w410 w425 w438 w449]
          tunnel: [w407 w417 w427 w441 w446] -> w390
          tunnel: w383 -> [_ w412 w423 w437 _]
          tunnel: w382 -> [_ w411 w422 w436 _]
          frame 0, Default {
          }
          frame 1, 131 {
            n212 = Unbundle By Name(w410) -> ("data.TP.TP.alarm_step"=w409:dbl)
            n213 = Unbundle By Name(w419) -> ("总磷控温温度1"=w418:sgl, "营养盐控温温度2"=w414:sgl)
            n214 = Select(t=w411, s=w412, f=w409) -> (s? t:f=w408:dbl)
            n215 = global read "VAR总磷总氮全局变量.vi" "总磷关键参数"() -> (w416:T20)
            n216 = Unbundle By Name(w416) -> ("消解温度"=w415:sgl)
            n217 = Bundle By Name(cluster=w410, "data.TP.TP.alarm_step"=w408, "data.TP.TP.digestion_temperature"=w418, "data.TP.TP.constant_temperature"=w415, "data.TP.TP.syringe_temperature"=w414, "data.TP.启用"=TRUE) -> (w417:T18)
            "总磷状态告警区" <- w420
          }
          frame 2, 76 {
            n218 = Unbundle By Name(w425) -> ("data.TN.TN.alarm_step"=w424:dbl)
            n219 = Unbundle By Name(w432) -> ("总磷控温温度1"=w428:sgl, "营养盐控温温度2"=w430:sgl)
            n220 = Select(t=w422, s=w423, f=w424) -> (s? t:f=w421:dbl)
            n221 = global read "VAR总磷总氮全局变量.vi" "总氮关键参数"() -> (w431:T20)
            n222 = Unbundle By Name(w431) -> ("消解温度"=w429:sgl)
            n223 = Bundle By Name(cluster=w425, "data.TN.TN.alarm_step"=w421, "data.TN.TN.digestion_temperature"=w428, "data.TN.TN.constant_temperature"=w429, "data.TN.TN.syringe_temperature"=w430, "data.TN.启用"=TRUE) -> (w427:T18)
            "总氮状态告警区" <- w433
          }
          frame 3 {
            n224 = Unbundle By Name(w438) -> ("data.NH3.NH3.alarm_step"=w435:dbl)
            n225 = Unbundle By Name(w442) -> ("营养盐控温温度2"=w440:sgl)
            n226 = Select(t=w436, s=w437, f=w435) -> (s? t:f=w434:dbl)
            n227 = Bundle By Name(cluster=w438, "data.NH3.NH3.alarm_step"=w434, "data.NH3.NH3.syringe_temperature"=w440, "data.NH3.启用"=TRUE) -> (w441:T18)
            "氨氮状态告警区" <- w443
          }
          frame 22 {
            n228 = Unbundle By Name(w448) -> ("营养盐控温温度2"=w447:sgl)
            n229 = global read "VAR总磷总氮全局变量.vi" "波形图-消解温度"() -> (w444:sgl[])
            n230 = Bundle By Name(cluster=w449, "data.CODCr.CODCr.temperature_curve"=w444, "data.CODCr.CODCr.reagent_sensor"=w447, "data.CODCr.启用"=TRUE) -> (w446:T18)
            "COD状态告警区" <- w450
          }
        }
        n231 = global write "工况数据接口全局.vi" "data"(w390) -> ()
      }
      frame "读关键参数区" {
        n232 = Variant To Data(type=u8 1 ("Slave ID"), Variant=w458) -> (data=w452:u8)  [unwired: 1 in, 1 out]
        n233 = property class="MB_Master"(reference=w461, error in=w462, "Properties:Slave ID"=w452) -> (reference out=w460:refnum<class "MB_Master.lvclass">, error out=w459:errorcluster)
        n234 = call "id参数转换.vi"("id"=w452) -> ("数组资源索引"=w451:i32)  [unwired: 9 in, 1 out]
        n235 = call <vilib>:"Read Holding Registers.vi"("error in (no error)"=w459, "quantity"=u16 56, "starting address"=u16 4256, "MB session in"=w460) -> ("error out"=w466:errorcluster, "Registers"=w456:u16[], "MB session out"=w465:refnum<class "MB_Master.lvclass">)  [unwired: 5 in]
        n236 = global read "VAR总磷总氮全局变量.vi" "关键参数区数组"() -> (w455:T6)
        n237 = call "关键参数区.vi"("数组"=w456) -> ("关键参数区"=w454:T3)  [unwired: 10 in]
        "关键参数区" <- w454
        n238 = global write "VAR总磷总氮全局变量.vi" "关键参数区"(w454) -> ()
        n239 = Replace Array Subset(array=w455, new element=w454, index=w451) -> (w453:T6)
        n240 = global write "VAR总磷总氮全局变量.vi" "关键参数区数组"(w453) -> ()
      }
      frame "shutdown" {
        n241 = call-dynamic "Close Session.vi"("error in (no error)"=w469, "MB session in"=w467) -> ("error out"=w468:errorcluster)  [unwired: 9 in]
        n242 = Flush Queue(queue=w471) -> (queue out=w470:refnum<queue>)  [unwired: 1 in, 2 out]
        n243 = Release Queue(queue=w470) -> ()  [unwired: 2 in, 3 out]
      }
    }
    n244 = global write "VAR总磷总氮全局变量.vi" "MB session in"(w186) -> ()
    n245 = Unbundle By Name(w192) -> ("status"=w189:bool)
    n246 = Not(x=w189) -> (.not. x?=w191:bool)
    "status" <- w191
    n247 = call <vilib>:"Boolean Crossing PtByPt.vi"("direction"=enum16{"either", "false-true", "true-false"}."false-true", "input"=w189) -> ("crossing"=w188:bool)  [unwired: 1 in]
    n248 = case shown="False" w188 {
      tunnel: [u16 0 ("告警代码") u16 999 ("告警代码")] -> w185
      frame False {
      }
      frame True {
      }
    }
    n249 = global write "VAR总磷总氮全局变量.vi" "通讯状态"(w191) -> ()
    n250 = call "告警码字段定义.vi"("id"=w184, "告警代码"=w185) -> ()  [unwired: 9 in, 1 out]
  }
  n251 = while {
    tunnel: w35 -> [w483]
    tunnel: w34 -> [w482]
    tunnel: w33 -> [w481]
    tunnel: w32 -> [w480]
    tunnel: w31 -> [w479]
    tunnel: w30 -> [w478]
    tunnel: w29 -> [w477]
    tunnel: w28 -> [w476]
    tunnel: w27 -> [w475]
    tunnel: w26 -> [w474]
    stop <- FALSE stop-if-true
    n252 = global read "model config var.vi" "启动队列名称"() -> (w486:cluster{"String":string, "Value":u16}[])
    n253 = Wait (ms)(milliseconds to wait=u32 1000 ("等待时间（毫秒）")) -> ()  [unwired: 1 out]
    n254 = global read "VAR总磷总氮全局变量.vi" "固件版本号"() -> (w473:string)
    n255 = for {
      tunnel: w486 -> [w499] mode=indexing
      tunnel: w483 -> [w497]
      tunnel: w482 -> [w496]
      tunnel: w481 -> [w495]
      tunnel: w480 -> [w494]
      tunnel: w479 -> [w493]
      tunnel: w478 -> [w492]
      tunnel: w477 -> [w491]
      tunnel: w476 -> [w490]
      tunnel: w475 -> [w489]
      tunnel: w474 -> [w488]
      tunnel: w473 -> [w487]
      n256 = Unbundle By Name(w499) -> ("Value"=w498:u16)
      n257 = case shown="1" w498 {
        tunnel: w497 -> [_ _ _ _ w586 _]
        tunnel: w496 -> [_ _ _ _ w585 _]
        tunnel: w495 -> [_ _ _ w565 _ _]
        tunnel: w494 -> [_ _ _ w564 _ _]
        tunnel: w493 -> [w502 _ _ _ _ _]
        tunnel: w492 -> [w501 _ _ _ _ _]
        tunnel: w491 -> [_ w523 _ _ _ _]
        tunnel: w490 -> [_ w522 _ _ _ _]
        tunnel: w489 -> [_ _ w544 _ _ _]
        tunnel: w488 -> [_ _ w543 _ _ _]
        tunnel: w487 -> [w500 w521 w542 w563 w584 _]
        frame 1 {
          n258 = Get Queue Status(queue=w502) -> (queue out=w505:refnum<queue>, # elements in queue=w504:i32)  [unwired: 2 in, 6 out]
          n259 = Equal To 0?(x=w504) -> (x = 0?=w503:bool)
          n260 = case shown="True" w503 {
            tunnel: w501 -> [_ w517]
            tunnel: w505 -> [_ w518]
            tunnel: w500 -> [_ w506]
            frame False {
            }
            frame True {
              w508 = u16 1 items=["总磷"=1, "总氮"=2, "氨氮"=3, "磷酸盐"=4, "硝氮"=5, "亚硝氮"=6, "硅酸盐"=7, "硫化物"=8, "CODCr"=22]
              n261 = Unbundle By Name(w517) -> ("关键参数"=w515:T21)
              n262 = global read "VAR总磷总氮全局变量.vi" "总磷关键参数"() -> (w516:T20)
              n263 = global read "VAR总磷总氮全局变量.vi" "状态告警区数组"() -> (w510:T7)
              n264 = global read "VAR总磷总氮全局变量.vi" "平台试剂余量百分比"() -> (w520:sgl)
              n265 = call "id参数转换.vi"("id"=w508) -> ("数组资源索引"=w509:i32)  [unwired: 9 in, 1 out]
              n266 = call "转换关键参数(子VI).vi"("参数"=w508, "总磷关键参数"=w516, "关键参数输入"=w515) -> ("关键参数输出"=w514:T21)  [unwired: 8 in]
              n267 = global read "VAR总磷总氮全局变量.vi" "总磷关键参数改变"() -> (w513:bool)
              n268 = global read "VAR总磷总氮全局变量.vi" "总磷校准信息改变"() -> (w511:bool)
              n269 = global read "VAR总磷总氮全局变量.vi" "总磷校准信息"() -> (w512:T22)
              n270 = Index Array(array=w510, index=w509) -> (element=w507:T4)
              n271 = Bundle By Name(cluster=w517, "状态告警区"=w507, "平台试剂余量百分比"=w520, "关键参数"=w514, "关键参数改变"=w513, "校准信息"=w512, "校准信息改变"=w511, "固件版本号"=w506) -> (w519:T13)
              n272 = Enqueue Element(queue=w518, element=w519) -> ()  [unwired: 2 in, 3 out]
            }
          }
        }
        frame 2 {
          n273 = Get Queue Status(queue=w523) -> (queue out=w526:refnum<queue>, # elements in queue=w525:i32)  [unwired: 2 in, 6 out]
          n274 = Equal To 0?(x=w525) -> (x = 0?=w524:bool)
          n275 = case shown="True" w524 {
            tunnel: w526 -> [_ w539]
            tunnel: w522 -> [_ w537]
            tunnel: w521 -> [_ w527]
            frame False {
            }
            frame True {
              w529 = u16 2 items=["总磷"=1, "总氮"=2, "氨氮"=3, "磷酸盐"=4, "硝氮"=5, "亚硝氮"=6, "硅酸盐"=7, "硫化物"=8, "CODCr"=22]
              n276 = Unbundle By Name(w537) -> ("关键参数"=w536:T21)
              n277 = global read "VAR总磷总氮全局变量.vi" "总氮关键参数"() -> (w538:T20)
              n278 = global read "VAR总磷总氮全局变量.vi" "状态告警区数组"() -> (w530:T7)
              n279 = global read "VAR总磷总氮全局变量.vi" "平台试剂余量百分比"() -> (w541:sgl)
              n280 = call "id参数转换.vi"("id"=w529) -> ("数组资源索引"=w531:i32)  [unwired: 9 in, 1 out]
              n281 = call "转换关键参数(子VI).vi"("参数"=w529, "总磷关键参数"=w538, "关键参数输入"=w536) -> ("关键参数输出"=w535:T21)  [unwired: 8 in]
              n282 = global read "VAR总磷总氮全局变量.vi" "总氮关键参数改变"() -> (w534:bool)
              n283 = global read "VAR总磷总氮全局变量.vi" "总氮校准信息改变"() -> (w532:bool)
              n284 = global read "VAR总磷总氮全局变量.vi" "总氮校准信息"() -> (w533:T22)
              n285 = Index Array(array=w530, index=w531) -> (element=w528:T4)
              n286 = Bundle By Name(cluster=w537, "状态告警区"=w528, "平台试剂余量百分比"=w541, "关键参数"=w535, "关键参数改变"=w534, "校准信息"=w533, "校准信息改变"=w532, "固件版本号"=w527) -> (w540:T12)
              n287 = Enqueue Element(queue=w539, element=w540) -> ()  [unwired: 2 in, 3 out]
            }
          }
        }
        frame 3 {
          (unwired) FALSE
          n288 = Get Queue Status(queue=w544) -> (queue out=w546:refnum<queue>, # elements in queue=w547:i32)  [unwired: 2 in, 6 out]
          n289 = Equal To 0?(x=w547) -> (x = 0?=w545:bool)
          n290 = case shown="True" w545 {
            tunnel: w546 -> [_ w560]
            tunnel: w543 -> [_ w559]
            tunnel: w542 -> [_ w548]
            frame False {
            }
            frame True {
              w550 = u16 3 items=["总磷"=1, "总氮"=2, "氨氮"=3, "磷酸盐"=4, "硝氮"=5, "亚硝氮"=6, "硅酸盐"=7, "硫化物"=8, "CODCr"=22]
              n291 = Unbundle By Name(w559) -> ("关键参数"=w558:T21)
              n292 = global read "VAR总磷总氮全局变量.vi" "氨氮关键参数"() -> (w556:T20)
              n293 = global read "VAR总磷总氮全局变量.vi" "状态告警区数组"() -> (w551:T7)
              n294 = global read "VAR总磷总氮全局变量.vi" "平台试剂余量百分比"() -> (w562:sgl)
              n295 = call "id参数转换.vi"("id"=w550) -> ("数组资源索引"=w552:i32)  [unwired: 9 in, 1 out]
              n296 = call "转换关键参数(子VI).vi"("参数"=w550, "总磷关键参数"=w556, "关键参数输入"=w558) -> ("关键参数输出"=w557:T21)  [unwired: 8 in]
              n297 = global read "VAR总磷总氮全局变量.vi" "氨氮关键参数改变"() -> (w555:bool)
              n298 = global read "VAR总磷总氮全局变量.vi" "氨氮校准信息改变"() -> (w553:bool)
              n299 = global read "VAR总磷总氮全局变量.vi" "氨氮校准信息"() -> (w554:T22)
              n300 = Index Array(array=w551, index=w552) -> (element=w549:T4)
              n301 = Bundle By Name(cluster=w559, "状态告警区"=w549, "平台试剂余量百分比"=w562, "关键参数"=w557, "关键参数改变"=w555, "校准信息"=w554, "校准信息改变"=w553, "固件版本号"=w548) -> (w561:T11)
              n302 = Enqueue Element(queue=w560, element=w561) -> ()  [unwired: 2 in, 3 out]
            }
          }
        }
        frame 22 {
          n303 = Get Queue Status(queue=w565) -> (queue out=w567:refnum<queue>, # elements in queue=w568:i32)  [unwired: 2 in, 6 out]
          n304 = Equal To 0?(x=w568) -> (x = 0?=w566:bool)
          n305 = case shown="True" w566 {
            tunnel: w567 -> [_ w581]
            tunnel: w564 -> [_ w580]
            tunnel: w563 -> [_ w569]
            frame False {
            }
            frame True {
              w571 = u16 22 items=["总磷"=1, "总氮"=2, "氨氮"=3, "磷酸盐"=4, "硝氮"=5, "亚硝氮"=6, "硅酸盐"=7, "硫化物"=8, "CODCr"=22]
              n306 = Unbundle By Name(w580) -> ("关键参数"=w579:T21)
              n307 = global read "VAR总磷总氮全局变量.vi" "CODcr关键参数"() -> (w578:T20)
              n308 = global read "VAR总磷总氮全局变量.vi" "状态告警区数组"() -> (w572:T7)
              n309 = global read "VAR总磷总氮全局变量.vi" "CODCr关键参数改变"() -> (w576:bool)
              n310 = global read "VAR总磷总氮全局变量.vi" "CODCr校准信息改变"() -> (w574:bool)
              n311 = global read "VAR总磷总氮全局变量.vi" "平台试剂余量百分比"() -> (w583:sgl)
              n312 = call "id参数转换.vi"("id"=w571) -> ("数组资源索引"=w573:i32)  [unwired: 9 in, 1 out]
              n313 = call "转换关键参数(子VI).vi"("参数"=w571, "总磷关键参数"=w578, "关键参数输入"=w579) -> ("关键参数输出"=w577:T21)  [unwired: 8 in]
              n314 = global read "VAR总磷总氮全局变量.vi" "CODCr校准信息"() -> (w575:T22)
              n315 = Index Array(array=w572, index=w573) -> (element=w570:T4)
              n316 = Bundle By Name(cluster=w580, "状态告警区"=w570, "平台试剂余量百分比"=w583, "关键参数"=w577, "关键参数改变"=w576, "校准信息"=w575, "校准信息改变"=w574, "固件版本号"=w569) -> (w582:T10)
              n317 = Enqueue Element(queue=w581, element=w582) -> ()  [unwired: 2 in, 3 out]
            }
          }
        }
        frame 21 {
          (unwired) FALSE
          n318 = Get Queue Status(queue=w586) -> (queue out=w588:refnum<queue>, # elements in queue=w589:i32)  [unwired: 2 in, 6 out]
          n319 = Equal To 0?(x=w589) -> (x = 0?=w587:bool)
          n320 = case shown="True" w587 {
            tunnel: w588 -> [_ w602]
            tunnel: w585 -> [_ w601]
            tunnel: w584 -> [_ w590]
            frame False {
            }
            frame True {
              w592 = u16 21 items=["总磷"=1, "总氮"=2, "氨氮"=3, "磷酸盐"=4, "硝氮"=5, "亚硝氮"=6, "硅酸盐"=7, "硫化物"=8, "CODMn"=21, "CODCr"=22, "氟化物"=50]
              n321 = Unbundle By Name(w601) -> ("关键参数"=w600:T21)
              n322 = global read "VAR总磷总氮全局变量.vi" "CODMn关键参数"() -> (w599:T20)
              n323 = global read "VAR总磷总氮全局变量.vi" "状态告警区数组"() -> (w593:T7)
              n324 = global read "VAR总磷总氮全局变量.vi" "CODmn关键参数改变"() -> (w597:bool)
              n325 = global read "VAR总磷总氮全局变量.vi" "CODMn校准信息改变"() -> (w595:bool)
              n326 = global read "VAR总磷总氮全局变量.vi" "平台试剂余量百分比"() -> (w604:sgl)
              n327 = call "id参数转换.vi"("id"=w592) -> ("数组资源索引"=w594:i32)  [unwired: 9 in, 1 out]
              n328 = call "转换关键参数(子VI).vi"("参数"=w592, "总磷关键参数"=w599, "关键参数输入"=w600) -> ("关键参数输出"=w598:T21)  [unwired: 8 in]
              n329 = global read "VAR总磷总氮全局变量.vi" "CODMn校准信息"() -> (w596:T22)
              n330 = Index Array(array=w593, index=w594) -> (element=w591:T4)
              n331 = Bundle By Name(cluster=w601, "状态告警区"=w591, "平台试剂余量百分比"=w604, "关键参数"=w598, "关键参数改变"=w597, "校准信息"=w596, "校准信息改变"=w595, "固件版本号"=w590) -> (w603:T10)
              n332 = Enqueue Element(queue=w602, element=w603) -> ()  [unwired: 2 in, 3 out]
            }
          }
        }
        frame Default {
        }
      }
    }
  }
